vi "Run.vi"(8 "error in (no error)":errorcluster, 11 "Channel in":refnum<class "Channel.lvclass">) -> (0 "error out":errorcluster, 3 "Channel out":refnum<class "Channel.lvclass">)   [LabVIEW 2018, in "Channel.lvclass"]
uses:
  Channel.lvclass
  Channel.lvclass/Channel.ctl
  Simulated_Image_Constructor/Simulated_Image_Constructor.lvclass/Simulated_Image_Constructor.ctl
  State Machine/State Machine.lvclass/State Machine.ctl
  Save Image/Save Image.lvclass/Save Image.ctl
  Simulated_CCD_Camera/Simulated_CCD_Camera.lvclass/Simulated_CCD_Camera.ctl
  Simulated_Cooler/Simulated_Cooler.lvclass/Simulated_Cooler.ctl
  Simulated_CCD_Camera/Simulated_CCD_Camera.lvclass
  State Machine/State Machine.lvclass
  Simulated_Cooler/Simulated_Cooler.lvclass
  Save Image/Save Image.lvclass
  Interface/Interface.lvclass
  RxTx/RxTx.lvclass
  Simulated_Image_Constructor/Simulated_Image_Constructor.lvclass
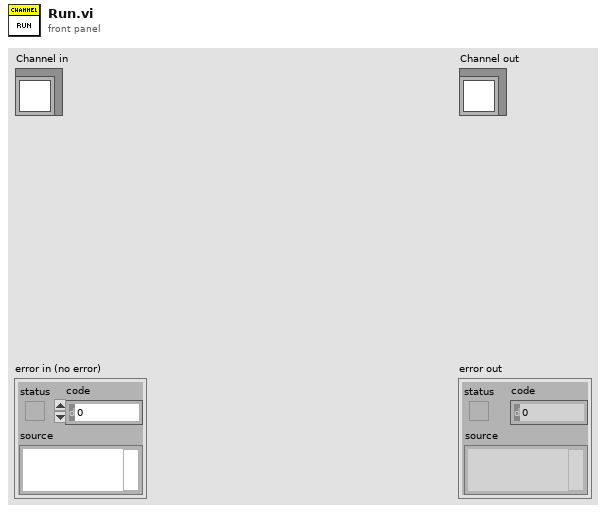
[diagram p1: front panel]
types:
  T1 = cluster{"Image Path":string, "Image Name":string, "Exposure Time":sgl, "Pre-amp gain":u8, "Readout Rate":u8, "EM Mode":u8, "EM Gain":u16, "Binning":u16, "Initial Line":u16, "Initial Cloumn":u16, "Final Line":u16, "Final Column":u16, "Kinetic Series Length":u32, "Shutter Mode":u8, "Cooler ON/OFF":u16, "Temperature":i8}
  T2 = cluster{"Exposure Time":sgl, "Pre-amp gain":u8, "Readout Rate":u8, "EM Mode":u8, "EM Gain":u16, "Binning":u16, "Initial Line":u16, "Initial Cloumn":u16, "Final Line":u16, "Final Column":u16, "Kinetic Series Length":u32, "Shutter Mode":u8, "Cooler ON/OFF":u8, "Temperature":i8, "Image Name":string, "Image Path":string, "Current Temperature":i16, "Temperatue Status":string, "Serial Number":u16, "#image":u32}
  T3 = cluster{"Exposure Time":sgl, "Pre-amp gain":u8, "Readout Rate":u8, "EM Mode":u8, "EM Gain":u16, "Binning":u16, "Initial Line":u16, "Initial Cloumn":u16, "Final Line":u16, "Final Column":u16, "Kinetic Series Length":u32, "Shutter Mode":u8, "Cooler ON/OFF":u16, "Temperature":i8, "Cubes":u32, "Trigger":u16}
  T4 = cluster{"Acquiring":bool, "Cube exposure time":sgl, "CCD status":string, "Frames done":u32, "Frame exposure time":dbl, "Initialization":bool, "Serial Number":u16}
  T5 = cluster{"Exposure Time":sgl, "EM Gain":u16, "Binning":u16, "Initial Line":u16, "Initial Cloumn":u16, "Final Line":u16, "Final Column":u16, "Kinetic Series Length":u32, "Shutter Mode":u8, "Pre-amp gain":u8, "Readout Rate":u8, "EM Mode":u8, "Trigger":u16, "Set Trigger":bool}
  T6 = cluster{"Initial Line":u16, "Initial Column":u16, "Final Line ":u16, "Final Column":u16, "Binning":u16, "Kinetic Series Length":u16, "Base Name":string, "Image Path":string}
  T7 = cluster{"Exposure Time":sgl, "Pre-amp gain":u8, "Readout Rate":u8, "EM Mode":u8, "EM Gain":u16, "Binning":u16, "Initial Line":u16, "Initial Cloumn":u16, "Final Line":u16, "Final Column":u16, "Kinetic Series Length":u32, "Shutter Mode":u8, "Cooler ON/OFF":u8, "Temperature":i8, "Image Name":string, "Image Path":string, "Current Temperature":i16, "Temperatue Status":string, "Serial Number":u16, " #image":u32}
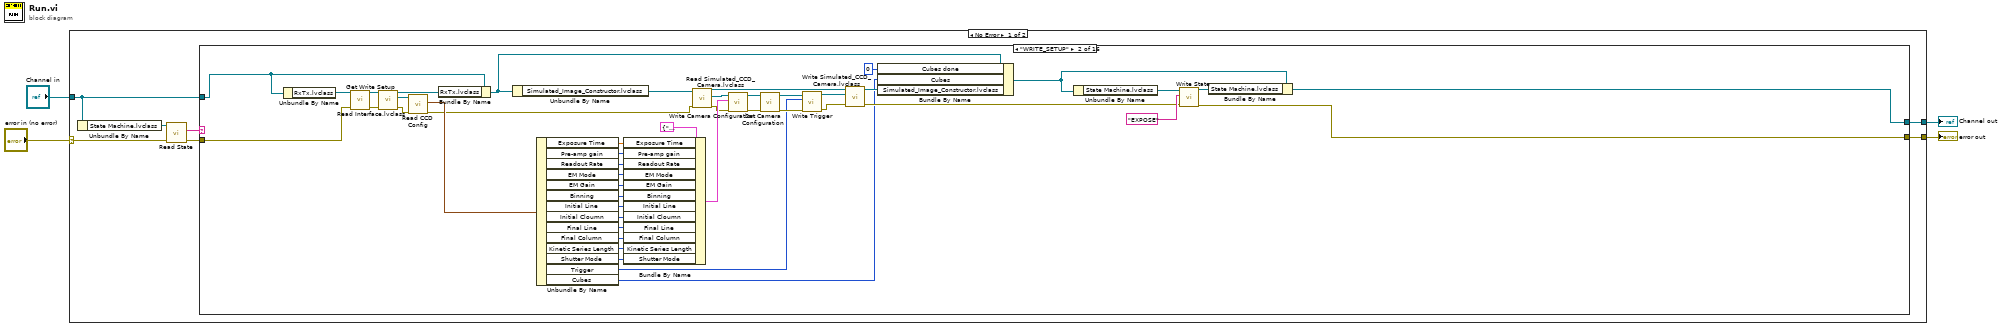
[diagram p0: block diagram]
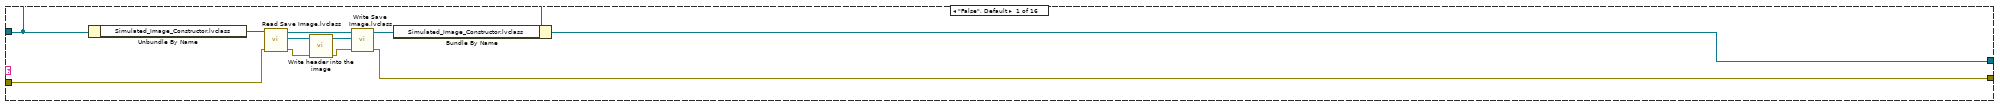
[diagram p2: hidden frame]
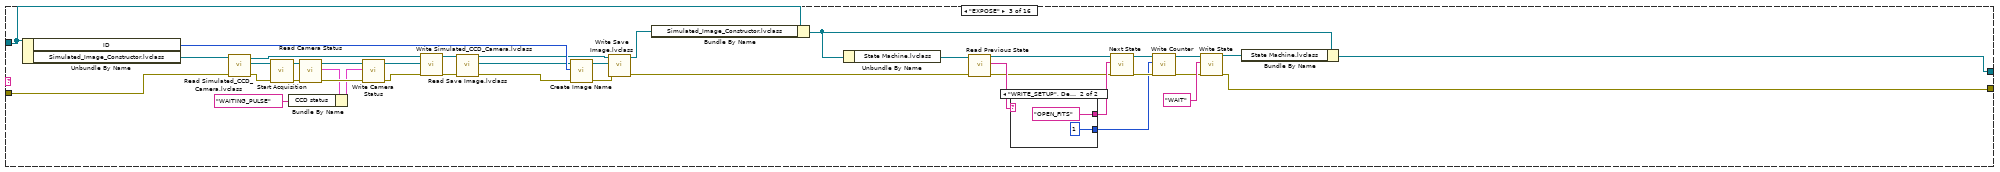
[diagram p3: hidden frame]
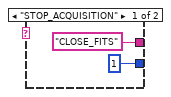
[diagram p4: hidden frame]
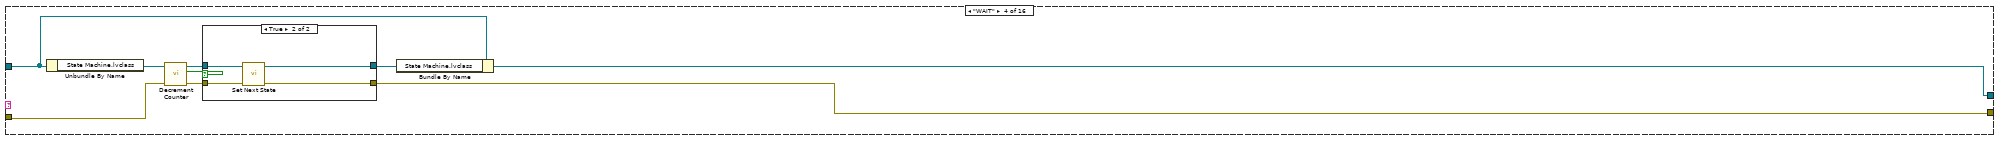
[diagram p5: hidden frame]
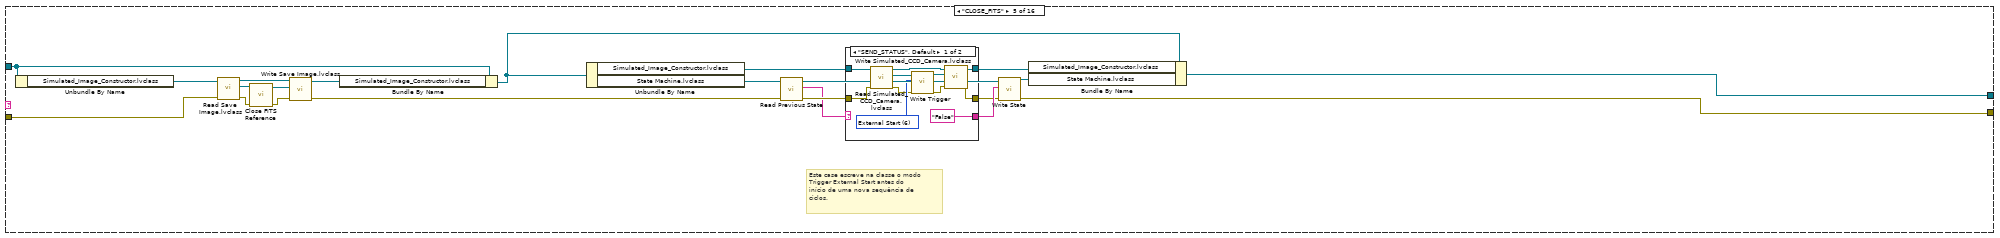
[diagram p7: hidden frame]
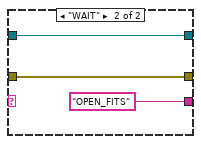
[diagram p8: hidden frame]
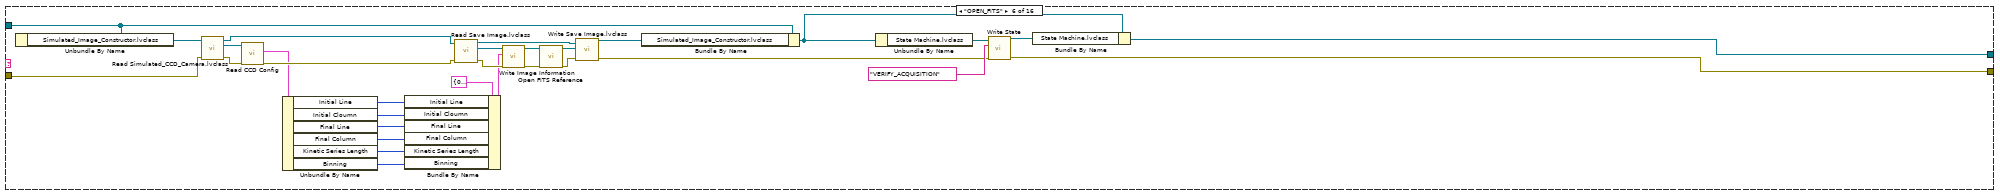
[diagram p9: hidden frame]
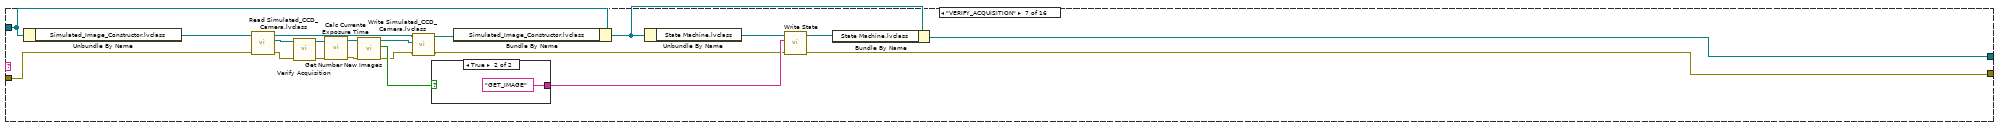
[diagram p10: hidden frame]
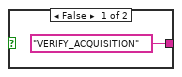
[diagram p11: hidden frame]
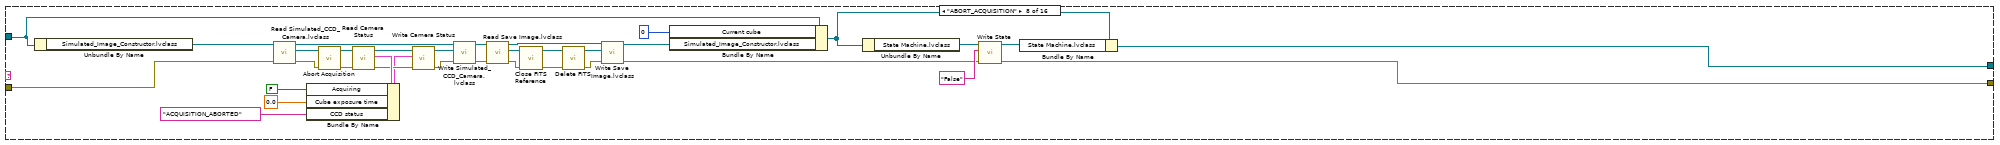
[diagram p12: hidden frame]
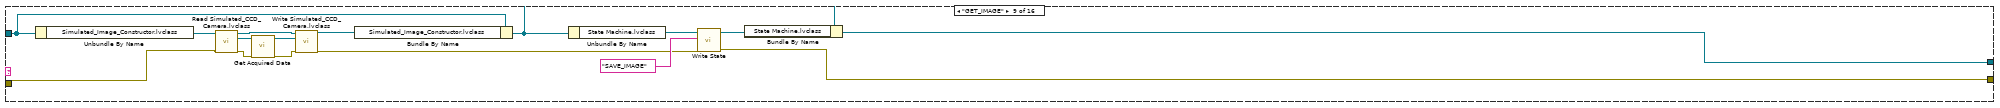
[diagram p13: hidden frame]
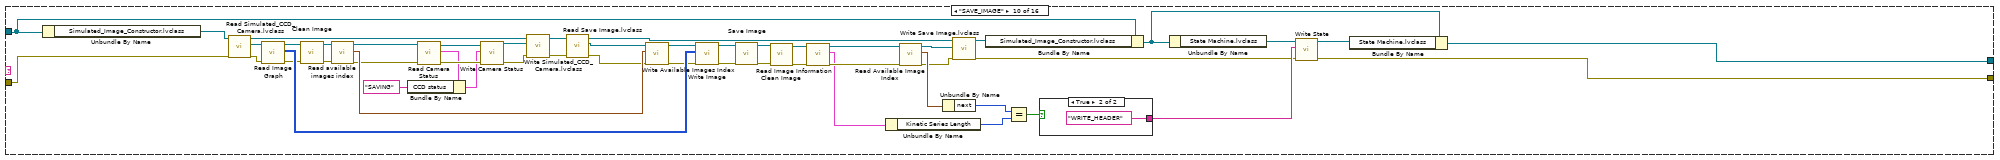
[diagram p14: hidden frame]
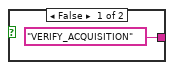
[diagram p15: hidden frame]
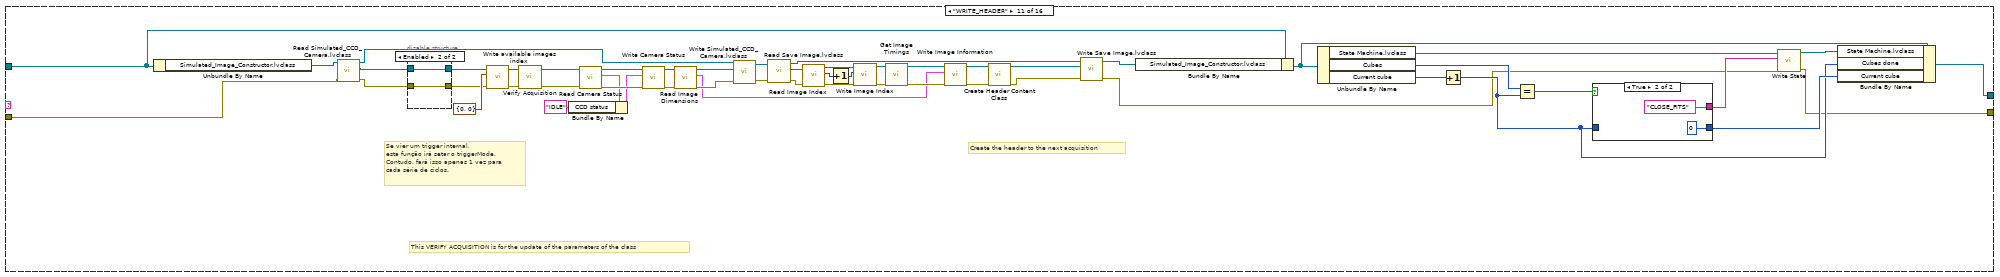
[diagram p16: hidden frame]
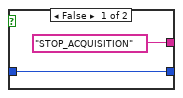
[diagram p17: hidden frame]
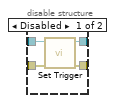
[diagram p18: hidden frame]
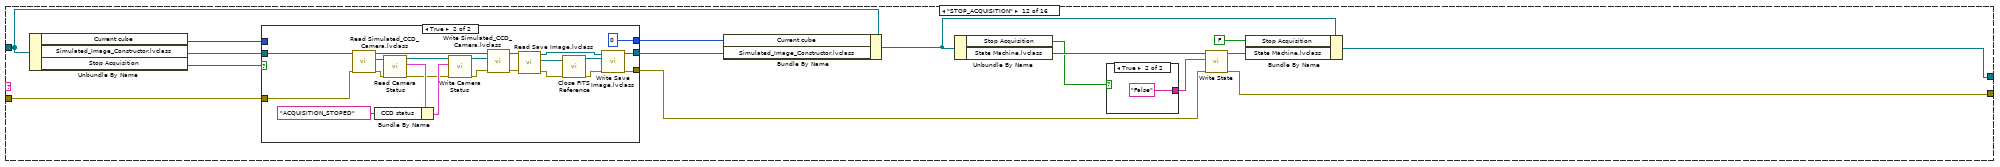
[diagram p19: hidden frame]
diagram:
  n1 = case shown="No Error" "error in (no error)" {
    selector: "error in (no error)" -> [w7 w1035]
    tunnel: [w11 w1035] -> w3
    tunnel: [w9 w1034] -> w1
    tunnel: "Channel in" -> [w10 w1034]
    frame No Error {
      n2 = Unbundle By Name(w10) -> ("State Machine.lvclass"=w8:refnum<class "State Machine.lvclass">)
      n3 = call-dynamic "Read State.vi"("error in (no error)"=w7, "State Machine in"=w8) -> ("error out"=w6:errorcluster, "State"=w5:string)  [unwired: 7 in, 1 out]
      n4 = case shown="\"WRITE_SETUP\"" w5 {
        tunnel: w6 -> [w14 w44 w83 w120 w130 w181 w202 w230 w259 w281 w346 w392 w428 w437 w836 w1017]
        tunnel: [w13 w39 w88 w117 w146 w190 w210 w248 w263 w296 w348 w396 w428 w430 w829 w1027] -> w11
        tunnel: [w21 w40 w85 w116 w148 w193 w213 w251 w268 w297 w349 w400 w429 w431 w830 w1028] -> w9
        tunnel: w10 -> [w22 w45 w108 w113 w149 w194 w215 w247 w267 w316 w373 w391 w429 w438 w837 w1033]
        frame "False", Default {
          n5 = Unbundle By Name(w22) -> ("Simulated_Image_Constructor.lvclass"=w20:refnum<class "Simulated_Image_Constructor.lvclass">)
          n6 = call "Read Save Image.lvclass.vi"("error in (no error)"=w14, "Image Constructor in"=w20) -> ("error out"=w16:errorcluster, "Save Image.lvclass"=w12:refnum<class "Save Image.lvclass">, "Image Constructor out"=w18:refnum<class "Simulated_Image_Constructor.lvclass">)  [unwired: 7 in]
          n7 = call "Write header into the image.vi"("error in (no error)"=w16, "Save Image in"=w12) -> ("error out"=w15:errorcluster, "Save Image out"=w19:refnum<class "Save Image.lvclass">)  [unwired: 8 in]
          n8 = call "Write Save Image.lvclass.vi"("error in (no error)"=w15, "Save Image.lvclass"=w19, "Image Constructor in"=w18) -> ("error out"=w13:errorcluster, "Image Constructor out"=w17:refnum<class "Simulated_Image_Constructor.lvclass">)  [unwired: 7 in]
          n9 = Bundle By Name(cluster=w22, "Simulated_Image_Constructor.lvclass"=w17) -> (w21:refnum<class "Channel.lvclass">)
        }
        frame "WRITE_SETUP" {
          n10 = Unbundle By Name(w45) -> ("RxTx.lvclass"=w62:refnum<class "RxTx.lvclass">)
          n11 = call "Get Write Setup.vi"("error in (no error)"=w44, "RxTx in"=w62) -> ("error out"=w63:errorcluster, "RxTx out"=w64:refnum<class "RxTx.lvclass">)  [unwired: 8 in]
          n12 = call "Read Interface.lvclass.vi"("error in (no error)"=w63, "RxTx in"=w64) -> ("error out"=w67:errorcluster, "Interface.lvclass"=w65:refnum<class "Interface.lvclass">, "RxTx out"=w66:refnum<class "RxTx.lvclass">)  [unwired: 7 in]
          n13 = call "Read CCD Config.vi"("error in (no error)"=w67, "Interface in"=w65) -> ("error out"=w31:errorcluster, "CCD Config"=w61:T3)  [unwired: 7 in, 1 out]
          n14 = Bundle By Name(cluster=w45, "RxTx.lvclass"=w66) -> (w60:refnum<class "Channel.lvclass">)
          n15 = Unbundle By Name(w60) -> ("Simulated_Image_Constructor.lvclass"=w30:refnum<class "Simulated_Image_Constructor.lvclass">)
          n16 = Unbundle By Name(w61) -> ("Exposure Time"=w35:sgl, "Pre-amp gain"=w49:u8, "Readout Rate"=w50:u8, "EM Mode"=w51:u8, "EM Gain"=w52:u16, "Binning"=w53:u16, "Initial Line"=w54:u16, "Initial Cloumn"=w55:u16, "Final Line"=w56:u16, "Final Column"=w57:u16, "Kinetic Series Length"=w34:u32, "Shutter Mode"=w58:u8, "Trigger"=w36:u16, "Cubes"=w24:u32)
          n17 = Bundle By Name(cluster=T1 {"Image Path"="", "Image Name"="Image", "Exposure Time"=0.1, "Pre-amp gain"=0, "Readout Rate"=0, "EM Mode"=0, "EM Gain"=2, "Binning"=1, "Initial Line"=1, "Initial Cloumn"=1, "Final Line"=1024, "Final Column"=1024, "Kinetic Series Length"=1, "Shutter Mode"=2, "Cooler ON/OFF"=0, "Temperature"=20} ("CCD Config"), "Exposure Time"=w35, "Pre-amp gain"=w49, "Readout Rate"=w50, "EM Mode"=w51, "EM Gain"=w52, "Binning"=w53, "Initial Line"=w54, "Initial Cloumn"=w55, "Final Line"=w56, "Final Column"=w57, "Kinetic Series Length"=w34, "Shutter Mode"=w58) -> (w59:T1)
          n18 = call "Read Simulated_CCD_Camera.lvclass.vi"("error in (no error)"=w31, "Image Constructor in"=w30) -> ("error out"=w32:errorcluster, "Simulated_CCD_Camera.lvclass"=w33:refnum<class "Simulated_CCD_Camera.lvclass">, "Image Constructor out"=w27:refnum<class "Simulated_Image_Constructor.lvclass">)  [unwired: 7 in]
          n19 = call-dynamic "Write Camera Configuration.vi"("error in (no error)"=w32, "CCD Config"=w59, "CCDCamera in"=w33) -> ("error out"=w47:errorcluster, "CCDCamera out"=w48:refnum<class "Simulated_CCD_Camera.lvclass">)  [unwired: 7 in]
          n20 = call-dynamic "Set Camera Configuration.vi"("error in (no error)"=w47, "CCDCamera in"=w48) -> ("error out"=w37:errorcluster, "CCDCamera out"=w38:refnum<class "Simulated_CCD_Camera.lvclass">)  [unwired: 8 in]
          n21 = call "Write Trigger.vi"("error in (no error)"=w37, "Trigger"=w36, "CCDCamera in"=w38) -> ("error out"=w29:errorcluster, "CCDCamera out"=w28:refnum<class "Simulated_CCD_Camera.lvclass">)  [unwired: 7 in]
          n22 = call "Write Simulated_CCD_Camera.lvclass.vi"("error in (no error)"=w29, "Simulated_CCD_Camera.lvclass"=w28, "Image Constructor in"=w27) -> ("error out"=w26:errorcluster, "Image Constructor out"=w25:refnum<class "Simulated_Image_Constructor.lvclass">)  [unwired: 7 in]
          n23 = Bundle By Name(cluster=w60, "Cubes done"=u16 0, "Cubes"=w24, "Simulated_Image_Constructor.lvclass"=w25) -> (w68:refnum<class "Channel.lvclass">)
          n24 = Unbundle By Name(w68) -> ("State Machine.lvclass"=w42:refnum<class "State Machine.lvclass">)
          n25 = call-dynamic "Write State.vi"("error in (no error)"=w26, "State"="EXPOSE", "State Machine in"=w42) -> ("error out"=w39:errorcluster, "State Machine out"=w43:refnum<class "State Machine.lvclass">)  [unwired: 7 in]
          n26 = Bundle By Name(cluster=w68, "State Machine.lvclass"=w43) -> (w40:refnum<class "Channel.lvclass">)
        }
        frame "EXPOSE" {
          n27 = Unbundle By Name(w108) -> ("ID"=w97:u8, "Simulated_Image_Constructor.lvclass"=w84:refnum<class "Simulated_Image_Constructor.lvclass">)
          n28 = call "Read Simulated_CCD_Camera.lvclass.vi"("error in (no error)"=w83, "Image Constructor in"=w84) -> ("error out"=w81:errorcluster, "Simulated_CCD_Camera.lvclass"=w82:refnum<class "Simulated_CCD_Camera.lvclass">, "Image Constructor out"=w80:refnum<class "Simulated_Image_Constructor.lvclass">)  [unwired: 7 in]
          n29 = call-dynamic "Start Acquisition.vi"("error in (no error)"=w81, "CCDCamera in"=w82) -> ("error out"=w106:errorcluster, "CCDCamera out"=w107:refnum<class "Simulated_CCD_Camera.lvclass">)  [unwired: 8 in]
          n30 = call "Read Camera Status.vi"("error in (no error)"=w106, "CCDCamera in"=w107) -> ("error out"=w104:errorcluster, "Camera Status"=w103:T4, "CCDCamera out"=w105:refnum<class "Simulated_CCD_Camera.lvclass">)  [unwired: 7 in]
          n31 = Bundle By Name(cluster=w103, "CCD status"="WAITING_PULSE" ("STATUS")) -> (w96:T4)
          n32 = call "Write Camera Status.vi"("error in (no error)"=w104, "Camera Status"=w96, "CCDCamera in"=w105) -> ("error out"=w71:errorcluster, "CCDCamera out"=w72:refnum<class "Simulated_CCD_Camera.lvclass">)  [unwired: 7 in]
          n33 = call "Write Simulated_CCD_Camera.lvclass.vi"("error in (no error)"=w71, "Simulated_CCD_Camera.lvclass"=w72, "Image Constructor in"=w80) -> ("error out"=w79:errorcluster, "Image Constructor out"=w78:refnum<class "Simulated_Image_Constructor.lvclass">)  [unwired: 7 in]
          n34 = call "Read Save Image.lvclass.vi"("error in (no error)"=w79, "Image Constructor in"=w78) -> ("error out"=w69:errorcluster, "Save Image.lvclass"=w70:refnum<class "Save Image.lvclass">, "Image Constructor out"=w75:refnum<class "Simulated_Image_Constructor.lvclass">)  [unwired: 7 in]
          n35 = call "Create Image Name.vi"("error in (no error)"=w69, "ID"=w97, "Save Image in"=w70) -> ("error out"=w77:errorcluster, "Save Image out"=w76:refnum<class "Save Image.lvclass">)  [unwired: 7 in]
          n36 = call "Write Save Image.lvclass.vi"("error in (no error)"=w77, "Save Image.lvclass"=w76, "Image Constructor in"=w75) -> ("error out"=w73:errorcluster, "Image Constructor out"=w74:refnum<class "Simulated_Image_Constructor.lvclass">)  [unwired: 7 in]
          n37 = Bundle By Name(cluster=w108, "Simulated_Image_Constructor.lvclass"=w74) -> (w86:refnum<class "Channel.lvclass">)
          n38 = Unbundle By Name(w86) -> ("State Machine.lvclass"=w101:refnum<class "State Machine.lvclass">)
          n39 = call-dynamic "Read Previous State.vi"("error in (no error)"=w73, "State Machine in"=w101) -> ("error out"=w99:errorcluster, "Previous State"=w100:string, "State Machine out"=w98:refnum<class "State Machine.lvclass">)  [unwired: 7 in]
          n40 = case shown="\"WRITE_SETUP\", Default" w100 {
            tunnel: ["CLOSE_FITS" "OPEN_FITS"] -> w102
            tunnel: [1 1] -> w89
            frame "STOP_ACQUISITION" {
            }
            frame "WRITE_SETUP", Default {
            }
          }
          n41 = call "Next State.vi"("error in (no error)"=w99, "New_State"=w102, "State Machine in"=w98) -> ("error out"=w90:errorcluster, "State Machine out"=w93:refnum<class "State Machine.lvclass">)  [unwired: 7 in]
          n42 = call "Write Counter.vi"("error in (no error)"=w90, "Counter"=w89, "State Machine in"=w93) -> ("error out"=w91:errorcluster, "State Machine out"=w92:refnum<class "State Machine.lvclass">)  [unwired: 7 in]
          n43 = call-dynamic "Write State.vi"("error in (no error)"=w91, "State"="WAIT", "State Machine in"=w92) -> ("error out"=w88:errorcluster, "State Machine out"=w87:refnum<class "State Machine.lvclass">)  [unwired: 7 in]
          n44 = Bundle By Name(cluster=w86, "State Machine.lvclass"=w87) -> (w85:refnum<class "Channel.lvclass">)
        }
        frame "WAIT" {
          n45 = Unbundle By Name(w113) -> ("State Machine.lvclass"=w121:refnum<class "State Machine.lvclass">)
          n46 = call "Decrement Counter.vi"("error in (no error)"=w120, "State Machine in"=w121) -> ("error out"=w118:errorcluster, "counter = zero"=w119:bool, "State Machine out"=w115:refnum<class "State Machine.lvclass">)  [unwired: 7 in]
          n47 = case shown="True" w119 {
            tunnel: w118 -> [w122 w127]
            tunnel: [w122 w125] -> w117
            tunnel: w115 -> [w123 w126]
            tunnel: [w123 w124] -> w114
            frame False {
            }
            frame True {
              n48 = call "Set Next State.vi"("error in (no error)"=w127, "State Machine in"=w126) -> ("error out"=w125:errorcluster, "State Machine out"=w124:refnum<class "State Machine.lvclass">)  [unwired: 8 in]
            }
          }
          n49 = Bundle By Name(cluster=w113, "State Machine.lvclass"=w114) -> (w116:refnum<class "Channel.lvclass">)
        }
        frame "CLOSE_FITS" {
          # "Este case escreve na classe o modo\nTrigger External Start antes do \ninício de uma nova sequência de \nciclos."
          n50 = Unbundle By Name(w149) -> ("Simulated_Image_Constructor.lvclass"=w133:refnum<class "Simulated_Image_Constructor.lvclass">)
          n51 = call "Read Save Image.lvclass.vi"("error in (no error)"=w130, "Image Constructor in"=w133) -> ("error out"=w137:errorcluster, "Save Image.lvclass"=w136:refnum<class "Save Image.lvclass">, "Image Constructor out"=w132:refnum<class "Simulated_Image_Constructor.lvclass">)  [unwired: 7 in]
          n52 = call "Close FITS Reference.vi"("error in (no error)"=w137, "Save Image in"=w136) -> ("error out"=w135:errorcluster, "Save Image out"=w134:refnum<class "Save Image.lvclass">)  [unwired: 8 in]
          n53 = call "Write Save Image.lvclass.vi"("error in (no error)"=w135, "Save Image.lvclass"=w134, "Image Constructor in"=w132) -> ("error out"=w128:errorcluster, "Image Constructor out"=w131:refnum<class "Simulated_Image_Constructor.lvclass">)  [unwired: 7 in]
          n54 = Bundle By Name(cluster=w149, "Simulated_Image_Constructor.lvclass"=w131) -> (w145:refnum<class "Channel.lvclass">)
          n55 = Unbundle By Name(w145) -> ("Simulated_Image_Constructor.lvclass"=w141:refnum<class "Simulated_Image_Constructor.lvclass">, "State Machine.lvclass"=w143:refnum<class "State Machine.lvclass">)
          n56 = call-dynamic "Read Previous State.vi"("error in (no error)"=w128, "State Machine in"=w143) -> ("error out"=w139:errorcluster, "Previous State"=w129:string, "State Machine out"=w142:refnum<class "State Machine.lvclass">)  [unwired: 7 in]
          n57 = case shown="\"SEND_STATUS\", Default" w129 {
            tunnel: ["False" "OPEN_FITS"] -> w144
            tunnel: w141 -> [w156 w162]
            tunnel: [w154 w162] -> w140
            tunnel: w139 -> [w155 w161]
            tunnel: [w153 w161] -> w138
            frame "SEND_STATUS", Default {
              w159 = u16 6 items=["Internal", "External", "-", "-", "-", "-", "External Start"] ("Trigger")
              n58 = call "Read Simulated_CCD_Camera.lvclass.vi"("error in (no error)"=w155, "Image Constructor in"=w156) -> ("error out"=w158:errorcluster, "Simulated_CCD_Camera.lvclass"=w157:refnum<class "Simulated_CCD_Camera.lvclass">, "Image Constructor out"=w150:refnum<class "Simulated_Image_Constructor.lvclass">)  [unwired: 7 in]
              n59 = call "Write Trigger.vi"("error in (no error)"=w158, "Trigger"=w159, "CCDCamera in"=w157) -> ("error out"=w152:errorcluster, "CCDCamera out"=w151:refnum<class "Simulated_CCD_Camera.lvclass">)  [unwired: 7 in]
              n60 = call "Write Simulated_CCD_Camera.lvclass.vi"("error in (no error)"=w152, "Simulated_CCD_Camera.lvclass"=w151, "Image Constructor in"=w150) -> ("error out"=w153:errorcluster, "Image Constructor out"=w154:refnum<class "Simulated_Image_Constructor.lvclass">)  [unwired: 7 in]
            }
            frame "WAIT" {
            }
          }
          n61 = call-dynamic "Write State.vi"("error in (no error)"=w138, "State"=w144, "State Machine in"=w142) -> ("error out"=w146:errorcluster, "State Machine out"=w147:refnum<class "State Machine.lvclass">)  [unwired: 7 in]
          n62 = Bundle By Name(cluster=w145, "Simulated_Image_Constructor.lvclass"=w140, "State Machine.lvclass"=w147) -> (w148:refnum<class "Channel.lvclass">)
        }
        frame "OPEN_FITS" {
          n63 = Unbundle By Name(w194) -> ("Simulated_Image_Constructor.lvclass"=w182:refnum<class "Simulated_Image_Constructor.lvclass">)
          n64 = call "Read Simulated_CCD_Camera.lvclass.vi"("error in (no error)"=w181, "Image Constructor in"=w182) -> ("error out"=w179:errorcluster, "Simulated_CCD_Camera.lvclass"=w180:refnum<class "Simulated_CCD_Camera.lvclass">, "Image Constructor out"=w178:refnum<class "Simulated_Image_Constructor.lvclass">)  [unwired: 7 in]
          n65 = call "Read CCD Config.vi"("error in (no error)"=w179, "CCDCamera in"=w180) -> ("error out"=w177:errorcluster, "CCD Config"=w170:T5)  [unwired: 7 in, 1 out]
          n66 = Unbundle By Name(w170) -> ("Initial Line"=w169:u16, "Initial Cloumn"=w168:u16, "Final Line"=w167:u16, "Final Column"=w166:u16, "Kinetic Series Length"=w165:u32, "Binning"=w164:u16)
          n67 = Bundle By Name(cluster=T2 {"Exposure Time"=0.0, "Pre-amp gain"=0, "Readout Rate"=0, "EM Mode"=0, "EM Gain"=2, "Binning"=1, "Initial Line"=1, "Initial Cloumn"=1, "Final Line"=1024, "Final Column"=1024, "Kinetic Series Length"=0, "Shutter Mode"=0, "Cooler ON/OFF"=0, "Temperature"=20, "Image Name"="", "Image Path"="", "Current Temperature"=0, "Temperatue Status"="", "Serial Number"=0, "#image"=0} ("CCD Config"), "Initial Line"=w169, "Initial Cloumn"=w168, "Final Line"=w167, "Final Column"=w166, "Kinetic Series Length"=w165, "Binning"=w164) -> (w172:T2)
          n68 = call "Read Save Image.lvclass.vi"("error in (no error)"=w177, "Image Constructor in"=w178) -> ("error out"=w173:errorcluster, "Save Image.lvclass"=w174:refnum<class "Save Image.lvclass">, "Image Constructor out"=w185:refnum<class "Simulated_Image_Constructor.lvclass">)  [unwired: 7 in]
          n69 = call "Write Image Information.vi"("error in (no error)"=w173, "CCD Config"=w172, "Save Image in"=w174) -> ("error out"=w176:errorcluster, "Save Image out"=w175:refnum<class "Save Image.lvclass">)  [unwired: 7 in]
          n70 = call "Open FITS Reference.vi"("error in (no error)"=w176, "Save Image in"=w175) -> ("error out"=w187:errorcluster, "Save Image out"=w186:refnum<class "Save Image.lvclass">)  [unwired: 8 in]
          n71 = call "Write Save Image.lvclass.vi"("error in (no error)"=w187, "Save Image.lvclass"=w186, "Image Constructor in"=w185) -> ("error out"=w183:errorcluster, "Image Constructor out"=w184:refnum<class "Simulated_Image_Constructor.lvclass">)  [unwired: 7 in]
          n72 = Bundle By Name(cluster=w194, "Simulated_Image_Constructor.lvclass"=w184) -> (w189:refnum<class "Channel.lvclass">)
          n73 = Unbundle By Name(w189) -> ("State Machine.lvclass"=w191:refnum<class "State Machine.lvclass">)
          n74 = call-dynamic "Write State.vi"("error in (no error)"=w183, "State"="VERIFY_ACQUISITION", "State Machine in"=w191) -> ("error out"=w190:errorcluster, "State Machine out"=w192:refnum<class "State Machine.lvclass">)  [unwired: 7 in]
          n75 = Bundle By Name(cluster=w189, "State Machine.lvclass"=w192) -> (w193:refnum<class "Channel.lvclass">)
        }
        frame "VERIFY_ACQUISITION" {
          n76 = Unbundle By Name(w215) -> ("Simulated_Image_Constructor.lvclass"=w203:refnum<class "Simulated_Image_Constructor.lvclass">)
          n77 = call "Read Simulated_CCD_Camera.lvclass.vi"("error in (no error)"=w202, "Image Constructor in"=w203) -> ("error out"=w200:errorcluster, "Simulated_CCD_Camera.lvclass"=w201:refnum<class "Simulated_CCD_Camera.lvclass">, "Image Constructor out"=w198:refnum<class "Simulated_Image_Constructor.lvclass">)  [unwired: 7 in]
          n78 = call-dynamic "Verify Acquisition.vi"("error in (no error)"=w200, "CCDCamera in"=w201) -> ("error out"=w204:errorcluster, "CCDCamera out"=w205:refnum<class "Simulated_CCD_Camera.lvclass">)  [unwired: 7 in, 1 out]
          n79 = call-dynamic "Calc Currente Exposure Time.vi"("error in (no error)"=w204, "CCDCamera in"=w205) -> ("error out"=w206:errorcluster, "CCDCamera out"=w207:refnum<class "Simulated_CCD_Camera.lvclass">)  [unwired: 8 in]
          n80 = call-dynamic "Get Number New Images.vi"("error in (no error)"=w206, "CCDCamera in"=w207) -> ("error out"=w196:errorcluster, "New Images ?"=w208:bool, "CCDCamera out"=w195:refnum<class "Simulated_CCD_Camera.lvclass">)  [unwired: 7 in]
          n81 = call "Write Simulated_CCD_Camera.lvclass.vi"("error in (no error)"=w196, "Simulated_CCD_Camera.lvclass"=w195, "Image Constructor in"=w198) -> ("error out"=w197:errorcluster, "Image Constructor out"=w199:refnum<class "Simulated_Image_Constructor.lvclass">)  [unwired: 7 in]
          n82 = case shown="True" w208 {
            tunnel: ["VERIFY_ACQUISITION" "GET_IMAGE"] -> w209
            frame False {
            }
            frame True {
            }
          }
          n83 = Bundle By Name(cluster=w215, "Simulated_Image_Constructor.lvclass"=w199) -> (w214:refnum<class "Channel.lvclass">)
          n84 = Unbundle By Name(w214) -> ("State Machine.lvclass"=w212:refnum<class "State Machine.lvclass">)
          n85 = call-dynamic "Write State.vi"("error in (no error)"=w197, "State"=w209, "State Machine in"=w212) -> ("error out"=w210:errorcluster, "State Machine out"=w211:refnum<class "State Machine.lvclass">)  [unwired: 7 in]
          n86 = Bundle By Name(cluster=w214, "State Machine.lvclass"=w211) -> (w213:refnum<class "Channel.lvclass">)
        }
        frame "ABORT_ACQUISITION" {
          n87 = Unbundle By Name(w247) -> ("Simulated_Image_Constructor.lvclass"=w231:refnum<class "Simulated_Image_Constructor.lvclass">)
          n88 = call "Read Simulated_CCD_Camera.lvclass.vi"("error in (no error)"=w230, "Image Constructor in"=w231) -> ("error out"=w232:errorcluster, "Simulated_CCD_Camera.lvclass"=w233:refnum<class "Simulated_CCD_Camera.lvclass">, "Image Constructor out"=w227:refnum<class "Simulated_Image_Constructor.lvclass">)  [unwired: 7 in]
          n89 = call-dynamic "Abort Acquisition.vi"("error in (no error)"=w232, "CCDCamera in"=w233) -> ("error out"=w239:errorcluster, "CCDCamera out"=w240:refnum<class "Simulated_CCD_Camera.lvclass">)  [unwired: 8 in]
          n90 = call "Read Camera Status.vi"("error in (no error)"=w239, "CCDCamera in"=w240) -> ("error out"=w237:errorcluster, "Camera Status"=w244:T4, "CCDCamera out"=w238:refnum<class "Simulated_CCD_Camera.lvclass">)  [unwired: 7 in]
          n91 = Bundle By Name(cluster=w244, "Acquiring"=FALSE, "Cube exposure time"=sgl 0.0 ("Current exptime"), "CCD status"="ACQUISITION_ABORTED" ("STATUS")) -> (w236:T4)
          n92 = call "Write Camera Status.vi"("error in (no error)"=w237, "Camera Status"=w236, "CCDCamera in"=w238) -> ("error out"=w229:errorcluster, "CCDCamera out"=w228:refnum<class "Simulated_CCD_Camera.lvclass">)  [unwired: 7 in]
          n93 = call "Write Simulated_CCD_Camera.lvclass.vi"("error in (no error)"=w229, "Simulated_CCD_Camera.lvclass"=w228, "Image Constructor in"=w227) -> ("error out"=w226:errorcluster, "Image Constructor out"=w225:refnum<class "Simulated_Image_Constructor.lvclass">)  [unwired: 7 in]
          n94 = call "Read Save Image.lvclass.vi"("error in (no error)"=w226, "Image Constructor in"=w225) -> ("error out"=w224:errorcluster, "Save Image.lvclass"=w223:refnum<class "Save Image.lvclass">, "Image Constructor out"=w221:refnum<class "Simulated_Image_Constructor.lvclass">)  [unwired: 7 in]
          n95 = call "Close FITS Reference.vi"("error in (no error)"=w224, "Save Image in"=w223) -> ("error out"=w234:errorcluster, "Save Image out"=w235:refnum<class "Save Image.lvclass">)  [unwired: 8 in]
          n96 = call "Delete FITS.vi"("error in (no error)"=w234, "Save Image in"=w235) -> ("error out"=w220:errorcluster, "Save Image out"=w222:refnum<class "Save Image.lvclass">)  [unwired: 8 in]
          n97 = call "Write Save Image.lvclass.vi"("error in (no error)"=w220, "Save Image.lvclass"=w222, "Image Constructor in"=w221) -> ("error out"=w218:errorcluster, "Image Constructor out"=w219:refnum<class "Simulated_Image_Constructor.lvclass">)  [unwired: 7 in]
          n98 = Bundle By Name(cluster=w247, "Current cube"=0, "Simulated_Image_Constructor.lvclass"=w219) -> (w252:refnum<class "Channel.lvclass">)
          n99 = Unbundle By Name(w252) -> ("State Machine.lvclass"=w250:refnum<class "State Machine.lvclass">)
          n100 = call-dynamic "Write State.vi"("error in (no error)"=w218, "State"="False", "State Machine in"=w250) -> ("error out"=w248:errorcluster, "State Machine out"=w249:refnum<class "State Machine.lvclass">)  [unwired: 7 in]
          n101 = Bundle By Name(cluster=w252, "State Machine.lvclass"=w249) -> (w251:refnum<class "Channel.lvclass">)
        }
        frame "GET_IMAGE" {
          n102 = Unbundle By Name(w267) -> ("Simulated_Image_Constructor.lvclass"=w260:refnum<class "Simulated_Image_Constructor.lvclass">)
          n103 = call "Read Simulated_CCD_Camera.lvclass.vi"("error in (no error)"=w259, "Image Constructor in"=w260) -> ("error out"=w258:errorcluster, "Simulated_CCD_Camera.lvclass"=w261:refnum<class "Simulated_CCD_Camera.lvclass">, "Image Constructor out"=w256:refnum<class "Simulated_Image_Constructor.lvclass">)  [unwired: 7 in]
          n104 = call-dynamic "Get Acquired Data.vi"("error in (no error)"=w258, "CCDCamera in"=w261) -> ("error out"=w254:errorcluster, "CCDCamera out"=w255:refnum<class "Simulated_CCD_Camera.lvclass">)  [unwired: 8 in]
          n105 = call "Write Simulated_CCD_Camera.lvclass.vi"("error in (no error)"=w254, "Simulated_CCD_Camera.lvclass"=w255, "Image Constructor in"=w256) -> ("error out"=w253:errorcluster, "Image Constructor out"=w257:refnum<class "Simulated_Image_Constructor.lvclass">)  [unwired: 7 in]
          n106 = Bundle By Name(cluster=w267, "Simulated_Image_Constructor.lvclass"=w257) -> (w266:refnum<class "Channel.lvclass">)
          n107 = Unbundle By Name(w266) -> ("State Machine.lvclass"=w264:refnum<class "State Machine.lvclass">)
          n108 = call-dynamic "Write State.vi"("error in (no error)"=w253, "State"="SAVE_IMAGE", "State Machine in"=w264) -> ("error out"=w263:errorcluster, "State Machine out"=w265:refnum<class "State Machine.lvclass">)  [unwired: 7 in]
          n109 = Bundle By Name(cluster=w266, "State Machine.lvclass"=w265) -> (w268:refnum<class "Channel.lvclass">)
        }
        frame "SAVE_IMAGE" {
          n110 = Unbundle By Name(w316) -> ("Simulated_Image_Constructor.lvclass"=w282:refnum<class "Simulated_Image_Constructor.lvclass">)
          n111 = call "Read Simulated_CCD_Camera.lvclass.vi"("error in (no error)"=w281, "Image Constructor in"=w282) -> ("error out"=w284:errorcluster, "Simulated_CCD_Camera.lvclass"=w283:refnum<class "Simulated_CCD_Camera.lvclass">, "Image Constructor out"=w280:refnum<class "Simulated_Image_Constructor.lvclass">)  [unwired: 7 in]
          n112 = call "Read Image Graph.vi"("error in (no error)"=w284, "CCDCamera in"=w283) -> ("error out"=w317:errorcluster, "Image Graph"=w319:u16[][][], "CCDCamera out"=w318:refnum<class "Simulated_CCD_Camera.lvclass">)  [unwired: 7 in]
          n113 = call "Clean Image.vi"("error in (no error)"=w317, "CCDCamera in"=w318) -> ("error out"=w310:errorcluster, "CCDCamera out"=w311:refnum<class "Simulated_CCD_Camera.lvclass">)  [unwired: 8 in]
          n114 = call "Read available images index.vi"("error in (no error)"=w310, "CCDCamera in"=w311) -> ("error out"=w287:errorcluster, "available images index"=w295:cluster{"previous":u16, "next":u16}, "CCDCamera out"=w289:refnum<class "Simulated_CCD_Camera.lvclass">)  [unwired: 7 in]
          n115 = call "Read Camera Status.vi"("error in (no error)"=w287, "CCDCamera in"=w289) -> ("error out"=w291:errorcluster, "Camera Status"=w286:T4, "CCDCamera out"=w288:refnum<class "Simulated_CCD_Camera.lvclass">)  [unwired: 7 in]
          n116 = Bundle By Name(cluster=w286, "CCD status"="SAVING" ("STATUS")) -> (w285:T4)
          n117 = call "Write Camera Status.vi"("error in (no error)"=w291, "Camera Status"=w285, "CCDCamera in"=w288) -> ("error out"=w278:errorcluster, "CCDCamera out"=w279:refnum<class "Simulated_CCD_Camera.lvclass">)  [unwired: 7 in]
          n118 = call "Write Simulated_CCD_Camera.lvclass.vi"("error in (no error)"=w278, "Simulated_CCD_Camera.lvclass"=w279, "Image Constructor in"=w280) -> ("error out"=w277:errorcluster, "Image Constructor out"=w276:refnum<class "Simulated_Image_Constructor.lvclass">)  [unwired: 7 in]
          n119 = call "Read Save Image.lvclass.vi"("error in (no error)"=w277, "Image Constructor in"=w276) -> ("error out"=w275:errorcluster, "Save Image.lvclass"=w274:refnum<class "Save Image.lvclass">, "Image Constructor out"=w271:refnum<class "Simulated_Image_Constructor.lvclass">)  [unwired: 7 in]
          n120 = call "Write Available Images Index.vi"("error in (no error)"=w275, "available images index"=w295, "Save Image in"=w274) -> ("error out"=w309:errorcluster, "Save Image out"=w308:refnum<class "Save Image.lvclass">)  [unwired: 7 in]
          n121 = call "Write Image.vi"("error in (no error)"=w309, "Image"=w319, "Save Image in"=w308) -> ("error out"=w312:errorcluster, "Save Image out"=w313:refnum<class "Save Image.lvclass">)  [unwired: 7 in]
          n122 = call "Save Image.vi"("error in (no error)"=w312, "Save Image in"=w313) -> ("error out"=w314:errorcluster, "Save Image out"=w315:refnum<class "Save Image.lvclass">)  [unwired: 8 in]
          n123 = call "Clean Image.vi"("error in (no error)"=w314, "Save Image in"=w315) -> ("error out"=w307:errorcluster, "Save Image out"=w306:refnum<class "Save Image.lvclass">)  [unwired: 8 in]
          n124 = call "Read Image Information.vi"("error in (no error)"=w307, "Save Image in"=w306) -> ("error out"=w305:errorcluster, "Image Information"=w304:T6, "Save Image out"=w292:refnum<class "Save Image.lvclass">)  [unwired: 7 in]
          n125 = Unbundle By Name(w304) -> ("Kinetic Series Length"=w303:u16)
          n126 = call "Read Available Image Index.vi"("error in (no error)"=w305, "Save Image in"=w292) -> ("error out"=w272:errorcluster, "available images index"=w294:cluster{"previous":u16, "next":u16}, "Save Image out"=w270:refnum<class "Save Image.lvclass">)  [unwired: 7 in]
          n127 = Unbundle By Name(w294) -> ("next"=w293:u16)
          n128 = call "Write Save Image.lvclass.vi"("error in (no error)"=w272, "Save Image.lvclass"=w270, "Image Constructor in"=w271) -> ("error out"=w269:errorcluster, "Image Constructor out"=w273:refnum<class "Simulated_Image_Constructor.lvclass">)  [unwired: 7 in]
          n129 = Bundle By Name(cluster=w316, "Simulated_Image_Constructor.lvclass"=w273) -> (w299:refnum<class "Channel.lvclass">)
          n130 = Equal?(x=w293, y=w303) -> (x = y?=w302:bool)
          n131 = case shown="True" w302 {
            tunnel: ["VERIFY_ACQUISITION" "WRITE_HEADER"] -> w300
            frame False {
            }
            frame True {
            }
          }
          n132 = Unbundle By Name(w299) -> ("State Machine.lvclass"=w301:refnum<class "State Machine.lvclass">)
          n133 = call-dynamic "Write State.vi"("error in (no error)"=w269, "State"=w300, "State Machine in"=w301) -> ("error out"=w296:errorcluster, "State Machine out"=w298:refnum<class "State Machine.lvclass">)  [unwired: 7 in]
          n134 = Bundle By Name(cluster=w299, "State Machine.lvclass"=w298) -> (w297:refnum<class "Channel.lvclass">)
        }
        frame "WRITE_HEADER" {
          # "Create the header to the next acquisition"
          # "Se vier um trigger internal, \nesta função irá setar o triggerMode.\nContudo, fará isso apenas 1 vez para\ncada série de ciclos."
          # "This VERIFY ACQUISITION is for the update of the parameters of the class"
          n135 = Unbundle By Name(w373) -> ("Simulated_Image_Constructor.lvclass"=w347:refnum<class "Simulated_Image_Constructor.lvclass">)
          n136 = call "Read Simulated_CCD_Camera.lvclass.vi"("error in (no error)"=w346, "Image Constructor in"=w347) -> ("error out"=w361:errorcluster, "Simulated_CCD_Camera.lvclass"=w360:refnum<class "Simulated_CCD_Camera.lvclass">, "Image Constructor out"=w359:refnum<class "Simulated_Image_Constructor.lvclass">)  [unwired: 7 in]
          n137 = disable-structure shown="Enabled" {
            disable-tunnel: [w382 w384] -> w363
            disable-tunnel: [w381 w383] -> w362
            disable-tunnel: w360 -> [w380 w384]
            disable-tunnel: w361 -> [w379 w383]
            frame Disabled {
              n138 = call-dynamic "Set Trigger.vi"("error in (no error)"=w379, "CCDCamera in"=w380) -> ("error out"=w381:errorcluster, "CCDCamera out"=w382:refnum<class "Simulated_CCD_Camera.lvclass">)  [unwired: 8 in]
            }
            frame Enabled {
            }
          }
          n139 = call "Write available images index.vi"("error in (no error)"=w362, "available images index"=cluster{"previous":u16, "next":u16} {"previous"=0, "next"=0}, "CCDCamera in"=w363) -> ("error out"=w371:errorcluster, "CCDCamera out"=w372:refnum<class "Simulated_CCD_Camera.lvclass">)  [unwired: 7 in]
          n140 = call-dynamic "Verify Acquisition.vi"("error in (no error)"=w371, "CCDCamera in"=w372) -> ("error out"=w365:errorcluster, "CCDCamera out"=w366:refnum<class "Simulated_CCD_Camera.lvclass">)  [unwired: 7 in, 1 out]
          n141 = call "Read Camera Status.vi"("error in (no error)"=w365, "CCDCamera in"=w366) -> ("error out"=w369:errorcluster, "Camera Status"=w368:T4, "CCDCamera out"=w370:refnum<class "Simulated_CCD_Camera.lvclass">)  [unwired: 7 in]
          n142 = Bundle By Name(cluster=w368, "CCD status"="IDLE" ("STATUS")) -> (w367:T4)
          n143 = call "Write Camera Status.vi"("error in (no error)"=w369, "Camera Status"=w367, "CCDCamera in"=w370) -> ("error out"=w331:errorcluster, "CCDCamera out"=w332:refnum<class "Simulated_CCD_Camera.lvclass">)  [unwired: 7 in]
          n144 = call "Read Image Dimensions.vi"("error in (no error)"=w331, "CCDCamera in"=w332) -> ("error out"=w330:errorcluster, "CCD Config"=w326:T7, "CCDCamera out"=w329:refnum<class "Simulated_CCD_Camera.lvclass">)  [unwired: 7 in]
          n145 = call "Write Simulated_CCD_Camera.lvclass.vi"("error in (no error)"=w330, "Simulated_CCD_Camera.lvclass"=w329, "Image Constructor in"=w359) -> ("error out"=w335:errorcluster, "Image Constructor out"=w336:refnum<class "Simulated_Image_Constructor.lvclass">)  [unwired: 7 in]
          n146 = call "Read Save Image.lvclass.vi"("error in (no error)"=w335, "Image Constructor in"=w336) -> ("error out"=w339:errorcluster, "Save Image.lvclass"=w338:refnum<class "Save Image.lvclass">, "Image Constructor out"=w337:refnum<class "Simulated_Image_Constructor.lvclass">)  [unwired: 7 in]
          n147 = call "Read Image Index.vi"("error in (no error)"=w339, "Save Image in"=w338) -> ("error out"=w342:errorcluster, "Image Index"=w341:u16, "Save Image out"=w343:refnum<class "Save Image.lvclass">)  [unwired: 7 in]
          n148 = Increment(x=w341) -> (x+1=w340:u16)
          n149 = call "Write Image Index.vi"("error in (no error)"=w342, "Image Index"=w340, "Save Image in"=w343) -> ("error out"=w344:errorcluster, "Save Image out"=w345:refnum<class "Save Image.lvclass">)  [unwired: 7 in]
          n150 = call "Get Image Timings.vi"("error in (no error)"=w344, "Save Image in"=w345) -> ("error out"=w327:errorcluster, "Save Image out"=w328:refnum<class "Save Image.lvclass">)  [unwired: 8 in]
          n151 = call "Write Image Information.vi"("error in (no error)"=w327, "CCD Config"=w326, "Save Image in"=w328) -> ("error out"=w325:errorcluster, "Save Image out"=w323:refnum<class "Save Image.lvclass">)  [unwired: 7 in]
          n152 = call "Create Header Content Class.vi"("error in (no error)"=w325, "Save Image in"=w323) -> ("error out"=w324:errorcluster, "Save Image out"=w322:refnum<class "Save Image.lvclass">)  [unwired: 8 in]
          n153 = call "Write Save Image.lvclass.vi"("error in (no error)"=w324, "Save Image.lvclass"=w322, "Image Constructor in"=w337) -> ("error out"=w333:errorcluster, "Image Constructor out"=w334:refnum<class "Simulated_Image_Constructor.lvclass">)  [unwired: 7 in]
          n154 = Bundle By Name(cluster=w373, "Simulated_Image_Constructor.lvclass"=w334) -> (w350:refnum<class "Channel.lvclass">)
          n155 = Unbundle By Name(w350) -> ("State Machine.lvclass"=w354:refnum<class "State Machine.lvclass">, "Cubes"=w356:u16, "Current cube"=w353:u16)
          n156 = Increment(x=w353) -> (x+1=w351:u16)
          n157 = Equal?(x=w356, y=w351) -> (x = y?=w355:bool)
          n158 = case shown="True" w355 {
            tunnel: ["STOP_ACQUISITION" "CLOSE_FITS"] -> w357
            tunnel: [w375 u16 0 ("current image")] -> w352
            tunnel: w351 -> [w375 _]
            frame False {
            }
            frame True {
            }
          }
          n159 = call-dynamic "Write State.vi"("error in (no error)"=w333, "State"=w357, "State Machine in"=w354) -> ("error out"=w348:errorcluster, "State Machine out"=w358:refnum<class "State Machine.lvclass">)  [unwired: 7 in]
          n160 = Bundle By Name(cluster=w350, "State Machine.lvclass"=w358, "Cubes done"=w351, "Current cube"=w352) -> (w349:refnum<class "Channel.lvclass">)
        }
        frame "STOP_ACQUISITION" {
          n161 = Unbundle By Name(w391) -> ("Current cube"=w386:u16, "Simulated_Image_Constructor.lvclass"=w393:refnum<class "Simulated_Image_Constructor.lvclass">, "Stop Acquisition"=w387:bool)
          n162 = case shown="True" w387 {
            tunnel: w393 -> [w403 w417]
            tunnel: w392 -> [w402 w416]
            tunnel: [w403 w405] -> w390
            tunnel: [w402 w404] -> w388
            tunnel: w386 -> [w401 _]
            tunnel: [w401 0] -> w385
            frame False {
            }
            frame True {
              n163 = call "Read Simulated_CCD_Camera.lvclass.vi"("error in (no error)"=w416, "Image Constructor in"=w417) -> ("error out"=w419:errorcluster, "Simulated_CCD_Camera.lvclass"=w418:refnum<class "Simulated_CCD_Camera.lvclass">, "Image Constructor out"=w413:refnum<class "Simulated_Image_Constructor.lvclass">)  [unwired: 7 in]
              n164 = call "Read Camera Status.vi"("error in (no error)"=w419, "CCDCamera in"=w418) -> ("error out"=w423:errorcluster, "Camera Status"=w425:T4, "CCDCamera out"=w422:refnum<class "Simulated_CCD_Camera.lvclass">)  [unwired: 7 in]
              n165 = Bundle By Name(cluster=w425, "CCD status"="ACQUISITION_STOPED") -> (w424:T4)
              n166 = call "Write Camera Status.vi"("error in (no error)"=w423, "Camera Status"=w424, "CCDCamera in"=w422) -> ("error out"=w415:errorcluster, "CCDCamera out"=w414:refnum<class "Simulated_CCD_Camera.lvclass">)  [unwired: 7 in]
              n167 = call "Write Simulated_CCD_Camera.lvclass.vi"("error in (no error)"=w415, "Simulated_CCD_Camera.lvclass"=w414, "Image Constructor in"=w413) -> ("error out"=w412:errorcluster, "Image Constructor out"=w411:refnum<class "Simulated_Image_Constructor.lvclass">)  [unwired: 7 in]
              n168 = call "Read Save Image.lvclass.vi"("error in (no error)"=w412, "Image Constructor in"=w411) -> ("error out"=w409:errorcluster, "Save Image.lvclass"=w410:refnum<class "Save Image.lvclass">, "Image Constructor out"=w406:refnum<class "Simulated_Image_Constructor.lvclass">)  [unwired: 7 in]
              n169 = call "Close FITS Reference.vi"("error in (no error)"=w409, "Save Image in"=w410) -> ("error out"=w408:errorcluster, "Save Image out"=w407:refnum<class "Save Image.lvclass">)  [unwired: 8 in]
              n170 = call "Write Save Image.lvclass.vi"("error in (no error)"=w408, "Save Image.lvclass"=w407, "Image Constructor in"=w406) -> ("error out"=w404:errorcluster, "Image Constructor out"=w405:refnum<class "Simulated_Image_Constructor.lvclass">)  [unwired: 7 in]
            }
          }
          n171 = Bundle By Name(cluster=w391, "Current cube"=w385, "Simulated_Image_Constructor.lvclass"=w390) -> (w389:refnum<class "Channel.lvclass">)
          n172 = Unbundle By Name(w389) -> ("Stop Acquisition"=w395:bool, "State Machine.lvclass"=w398:refnum<class "State Machine.lvclass">)
          n173 = case shown="True" w395 {
            tunnel: ["EXPOSE" "False"] -> w394
            frame False {
            }
            frame True {
            }
          }
          n174 = call-dynamic "Write State.vi"("error in (no error)"=w388, "State"=w394, "State Machine in"=w398) -> ("error out"=w396:errorcluster, "State Machine out"=w397:refnum<class "State Machine.lvclass">)  [unwired: 7 in]
          n175 = Bundle By Name(cluster=w389, "Stop Acquisition"=FALSE, "State Machine.lvclass"=w397) -> (w400:refnum<class "Channel.lvclass">)
        }
        frame "N/A" {
        }
        frame "SET" {
          n176 = Unbundle By Name(w438) -> ("RxTx.lvclass"=w444:refnum<class "RxTx.lvclass">)
          n177 = call "Read Rx Value.vi"("error in (no error)"=w437, "RxTx in"=w444) -> ("error out"=w446:errorcluster, "Rx value"=w445:string, "RxTx out"=w447:refnum<class "RxTx.lvclass">)  [unwired: 7 in]
          n178 = case shown="\"READOUT\"" w445 {
            tunnel: [w450 w462 w490 w518 w541 w561 w582 w602 w620 w638 w649 w671 w686 w703 w718 w733 w756 w775 w796 w814 w816 w823] -> w443
            tunnel: w438 -> [w450 w463 w489 w517 w540 w560 w581 w601 w619 w637 w650 w670 w685 w702 w717 w732 w755 w774 w795 w813 w820 w823]
            tunnel: [w449 w451 w470 w503 w529 w544 w568 w591 w609 w627 w644 w657 w674 w687 w706 w721 w740 w763 w785 w797 w817 w825] -> w440
            tunnel: w446 -> [w449 w468 w488 w515 w539 w558 w580 w599 w617 w635 w655 w669 w683 w700 w715 w730 w754 w773 w792 w811 w821 w826]
            tunnel: w447 -> [_ w467 w487 w514 w538 w557 w579 w598 w616 w634 w654 w668 w684 w701 w716 w731 w753 w772 w793 w810 w822 w827]
            tunnel: ["INVALID_PARAMETER" "DONE" "DONE" "DONE" "DONE" "DONE" "DONE" "DONE" "DONE" "DONE" "DONE" "DONE" "DONE" "DONE" "DONE" "DONE" "DONE" "DONE" "DONE" "DONE" "DONE" "DONE"] -> w439
            frame "False", Default {
            }
            frame "EXPTIME" {
              n179 = call "Read Tx Value.vi"("error in (no error)"=w468, "RxTx in"=w467) -> ("error out"=w458:errorcluster, "Rx Value"=w466:string)  [unwired: 7 in, 1 out]
              n180 = Unbundle By Name(w463) -> ("Simulated_Image_Constructor.lvclass"=w459:refnum<class "Simulated_Image_Constructor.lvclass">)
              n181 = Fract/Exp String To Number(string=w466, default (0 dbl)=sgl 0.0) -> (number=w469:sgl)  [unwired: 2 in, 1 out]
              n182 = call "Read Simulated_CCD_Camera.lvclass.vi"("error in (no error)"=w458, "Image Constructor in"=w459) -> ("error out"=w457:errorcluster, "Simulated_CCD_Camera.lvclass"=w456:refnum<class "Simulated_CCD_Camera.lvclass">, "Image Constructor out"=w454:refnum<class "Simulated_Image_Constructor.lvclass">)  [unwired: 7 in]
              n183 = call "Write Exposure Time.vi"("error in (no error)"=w457, "Exposure Time"=w469, "CCDCamera in"=w456) -> ("error out"=w464:errorcluster, "CCDCamera out"=w465:refnum<class "Simulated_CCD_Camera.lvclass">)  [unwired: 7 in]
              n184 = call-dynamic "Set Exposure Time.vi"("error in (no error)"=w464, "CCDCamera in"=w465) -> ("error out"=w453:errorcluster, "CCDCamera out"=w452:refnum<class "Simulated_CCD_Camera.lvclass">)  [unwired: 8 in]
              n185 = call "Write Simulated_CCD_Camera.lvclass.vi"("error in (no error)"=w453, "Simulated_CCD_Camera.lvclass"=w452, "Image Constructor in"=w454) -> ("error out"=w451:errorcluster, "Image Constructor out"=w455:refnum<class "Simulated_Image_Constructor.lvclass">)  [unwired: 7 in]
              n186 = Bundle By Name(cluster=w463, "Simulated_Image_Constructor.lvclass"=w455) -> (w462:refnum<class "Channel.lvclass">)
            }
            frame "READOUT" {
              n187 = call "Read Tx Value.vi"("error in (no error)"=w488, "RxTx in"=w487) -> ("error out"=w477:errorcluster, "Rx Value"=w483:string)  [unwired: 7 in, 1 out]
              n188 = Unbundle By Name(w489) -> ("Simulated_Image_Constructor.lvclass"=w478:refnum<class "Simulated_Image_Constructor.lvclass">)
              n189 = call "Read Simulated_CCD_Camera.lvclass.vi"("error in (no error)"=w477, "Image Constructor in"=w478) -> ("error out"=w475:errorcluster, "Simulated_CCD_Camera.lvclass"=w476:refnum<class "Simulated_CCD_Camera.lvclass">, "Image Constructor out"=w472:refnum<class "Simulated_Image_Constructor.lvclass">)  [unwired: 7 in]
              n190 = call "Read EM Mode.vi"("error in (no error)"=w475, "CCDCamera in"=w476) -> ("error out"=w481:errorcluster, "EM Mode"=w484:u8, "CCDCamera out"=w480:refnum<class "Simulated_CCD_Camera.lvclass">)  [unwired: 7 in]
              n191 = case shown="1" w484 {
                tunnel: w483 -> [w492 w496]
                tunnel: [w491 w495] -> w482
                frame 0, Default {
                  n192 = case shown="\"0.1\"" w492 {
                    tunnel: [_ 0 1] -> w491
                    frame "False", Default {
                    }
                    frame "0.1" {
                    }
                    frame "1" {
                    }
                  }
                }
                frame 1 {
                  n193 = case shown="\"30\"" w496 {
                    tunnel: [_ 0 1 2 3] -> w495
                    frame "False", Default {
                    }
                    frame "30" {
                    }
                    frame "20" {
                    }
                    frame "10" {
                    }
                    frame "1" {
                    }
                  }
                }
              }
              n194 = call "Write Readout Rate.vi"("error in (no error)"=w481, "Readout Rate"=w482, "CCDCamera in"=w480) -> ("error out"=w485:errorcluster, "CCDCamera out"=w486:refnum<class "Simulated_CCD_Camera.lvclass">)  [unwired: 7 in]
              n195 = call-dynamic "Set HSS and EM Mode.vi"("error in (no error)"=w485, "CCDCamera in"=w486) -> ("error out"=w473:errorcluster, "CCDCamera out"=w474:refnum<class "Simulated_CCD_Camera.lvclass">)  [unwired: 8 in]
              n196 = call "Write Simulated_CCD_Camera.lvclass.vi"("error in (no error)"=w473, "Simulated_CCD_Camera.lvclass"=w474, "Image Constructor in"=w472) -> ("error out"=w470:errorcluster, "Image Constructor out"=w471:refnum<class "Simulated_Image_Constructor.lvclass">)  [unwired: 7 in]
              n197 = Bundle By Name(cluster=w489, "Simulated_Image_Constructor.lvclass"=w471) -> (w490:refnum<class "Channel.lvclass">)
            }
            frame "BINNING" {
              n198 = call "Read Tx Value.vi"("error in (no error)"=w515, "RxTx in"=w514) -> ("error out"=w508:errorcluster, "Rx Value"=w513:string)  [unwired: 7 in, 1 out]
              n199 = Unbundle By Name(w517) -> ("Simulated_Image_Constructor.lvclass"=w509:refnum<class "Simulated_Image_Constructor.lvclass">)
              n200 = Decimal String To Number(string=w513) -> (number=w516:i32)  [unwired: 2 in, 1 out]
              n201 = call "Read Simulated_CCD_Camera.lvclass.vi"("error in (no error)"=w508, "Image Constructor in"=w509) -> ("error out"=w507:errorcluster, "Simulated_CCD_Camera.lvclass"=w506:refnum<class "Simulated_CCD_Camera.lvclass">, "Image Constructor out"=w501:refnum<class "Simulated_Image_Constructor.lvclass">)  [unwired: 7 in]
              n202 = call "Write Binning.vi"("error in (no error)"=w507, "Binning"=w516, "CCDCamera in"=w506) -> ("error out"=w511:errorcluster, "CCDCamera out"=w512:refnum<class "Simulated_CCD_Camera.lvclass">)  [unwired: 7 in]
              n203 = call-dynamic "Set Image.vi"("error in (no error)"=w511, "CCDCamera in"=w512) -> ("error out"=w504:errorcluster, "CCDCamera out"=w505:refnum<class "Simulated_CCD_Camera.lvclass">)  [unwired: 8 in]
              n204 = call "Write Simulated_CCD_Camera.lvclass.vi"("error in (no error)"=w504, "Simulated_CCD_Camera.lvclass"=w505, "Image Constructor in"=w501) -> ("error out"=w503:errorcluster, "Image Constructor out"=w502:refnum<class "Simulated_Image_Constructor.lvclass">)  [unwired: 7 in]
              n205 = Bundle By Name(cluster=w517, "Simulated_Image_Constructor.lvclass"=w502) -> (w518:refnum<class "Channel.lvclass">)
            }
            frame "COOLER" {
              n206 = call "Read Tx Value.vi"("error in (no error)"=w539, "RxTx in"=w538) -> ("error out"=w523:errorcluster, "Rx Value"=w534:string)  [unwired: 7 in, 1 out]
              n207 = Unbundle By Name(w540) -> ("Simulated_Image_Constructor.lvclass"=w527:refnum<class "Simulated_Image_Constructor.lvclass">)
              n208 = call "Read Simulated_CCD_Camera.lvclass.vi"("error in (no error)"=w523, "Image Constructor in"=w527) -> ("error out"=w524:errorcluster, "Simulated_CCD_Camera.lvclass"=w525:refnum<class "Simulated_CCD_Camera.lvclass">, "Image Constructor out"=w526:refnum<class "Simulated_Image_Constructor.lvclass">)  [unwired: 7 in]
              n209 = case shown="\"OFFe\", Default" w534 {
                tunnel: [0 1] -> w533
                frame "OFFe", Default {
                }
                frame "ON" {
                }
              }
              n210 = call-dynamic "Read Cooler.lvclass.vi"("error in (no error)"=w524, "CCDCamera in"=w525) -> ("error out"=w536:errorcluster, "Simulated_Cooler.lvclass"=w537:refnum<class "Simulated_Cooler.lvclass">, "CCDCamera out"=w535:refnum<class "Simulated_CCD_Camera.lvclass">)  [unwired: 7 in]
              n211 = call "Write Cooler ON_OFF.vi"("error in (no error)"=w536, "Cooler ON/OFF"=w533, "Cooler in"=w537) -> ("error out"=w519:errorcluster, "Cooler out"=w522:refnum<class "Simulated_Cooler.lvclass">)  [unwired: 7 in]
              n212 = call-dynamic "Set Cooler ON - OFF.vi"("error in (no error)"=w519, "Cooler in"=w522) -> ("error out"=w520:errorcluster, "Cooler out"=w521:refnum<class "Simulated_Cooler.lvclass">)  [unwired: 8 in]
              n213 = call-dynamic "Write Cooler.lvclass.vi"("error in (no error)"=w520, "Simulated_Cooler.lvclass"=w521, "CCDCamera in"=w535) -> ("error out"=w530:errorcluster, "CCDCamera out"=w531:refnum<class "Simulated_CCD_Camera.lvclass">)  [unwired: 7 in]
              n214 = call "Write Simulated_CCD_Camera.lvclass.vi"("error in (no error)"=w530, "Simulated_CCD_Camera.lvclass"=w531, "Image Constructor in"=w526) -> ("error out"=w529:errorcluster, "Image Constructor out"=w528:refnum<class "Simulated_Image_Constructor.lvclass">)  [unwired: 7 in]
              n215 = Bundle By Name(cluster=w540, "Simulated_Image_Constructor.lvclass"=w528) -> (w541:refnum<class "Channel.lvclass">)
            }
            frame "EM_GAIN" {
              n216 = call "Read Tx Value.vi"("error in (no error)"=w558, "RxTx in"=w557) -> ("error out"=w551:errorcluster, "Rx Value"=w556:string)  [unwired: 7 in, 1 out]
              n217 = Unbundle By Name(w560) -> ("Simulated_Image_Constructor.lvclass"=w552:refnum<class "Simulated_Image_Constructor.lvclass">)
              n218 = Decimal String To Number(string=w556) -> (number=w559:i32)  [unwired: 2 in, 1 out]
              n219 = call "Read Simulated_CCD_Camera.lvclass.vi"("error in (no error)"=w551, "Image Constructor in"=w552) -> ("error out"=w550:errorcluster, "Simulated_CCD_Camera.lvclass"=w549:refnum<class "Simulated_CCD_Camera.lvclass">, "Image Constructor out"=w546:refnum<class "Simulated_Image_Constructor.lvclass">)  [unwired: 7 in]
              n220 = call "Write EM Gain.vi"("error in (no error)"=w550, "EM Gain"=w559, "CCDCamera in"=w549) -> ("error out"=w555:errorcluster, "CCDCamera out"=w554:refnum<class "Simulated_CCD_Camera.lvclass">)  [unwired: 7 in]
              n221 = call-dynamic "Set EM Gain.vi"("error in (no error)"=w555, "CCDCamera in"=w554) -> ("error out"=w547:errorcluster, "CCDCamera out"=w548:refnum<class "Simulated_CCD_Camera.lvclass">)  [unwired: 8 in]
              n222 = call "Write Simulated_CCD_Camera.lvclass.vi"("error in (no error)"=w547, "Simulated_CCD_Camera.lvclass"=w548, "Image Constructor in"=w546) -> ("error out"=w544:errorcluster, "Image Constructor out"=w545:refnum<class "Simulated_Image_Constructor.lvclass">)  [unwired: 7 in]
              n223 = Bundle By Name(cluster=w560, "Simulated_Image_Constructor.lvclass"=w545) -> (w561:refnum<class "Channel.lvclass">)
            }
            frame "EM_MODE" {
              n224 = call "Read Tx Value.vi"("error in (no error)"=w580, "RxTx in"=w579) -> ("error out"=w565:errorcluster, "Rx Value"=w578:string)  [unwired: 7 in, 1 out]
              n225 = Unbundle By Name(w581) -> ("Simulated_Image_Constructor.lvclass"=w566:refnum<class "Simulated_Image_Constructor.lvclass">)
              n226 = case shown="\"EM\"" w578 {
                tunnel: [1 0] -> w577
                frame "CONVENTIONAL", Default {
                }
                frame "EM" {
                }
              }
              n227 = call "Read Simulated_CCD_Camera.lvclass.vi"("error in (no error)"=w565, "Image Constructor in"=w566) -> ("error out"=w564:errorcluster, "Simulated_CCD_Camera.lvclass"=w563:refnum<class "Simulated_CCD_Camera.lvclass">, "Image Constructor out"=w562:refnum<class "Simulated_Image_Constructor.lvclass">)  [unwired: 7 in]
              n228 = call "Write EM Mode.vi"("error in (no error)"=w564, "EM Mode"=w577, "CCDCamera in"=w563) -> ("error out"=w573:errorcluster, "CCDCamera out"=w576:refnum<class "Simulated_CCD_Camera.lvclass">)  [unwired: 7 in]
              n229 = call "Write Readout Rate.vi"("error in (no error)"=w573, "Readout Rate"=0, "CCDCamera in"=w576) -> ("error out"=w574:errorcluster, "CCDCamera out"=w575:refnum<class "Simulated_CCD_Camera.lvclass">)  [unwired: 7 in]
              n230 = call-dynamic "Set HSS and EM Mode.vi"("error in (no error)"=w574, "CCDCamera in"=w575) -> ("error out"=w567:errorcluster, "CCDCamera out"=w570:refnum<class "Simulated_CCD_Camera.lvclass">)  [unwired: 8 in]
              n231 = call "Write Simulated_CCD_Camera.lvclass.vi"("error in (no error)"=w567, "Simulated_CCD_Camera.lvclass"=w570, "Image Constructor in"=w562) -> ("error out"=w568:errorcluster, "Image Constructor out"=w569:refnum<class "Simulated_Image_Constructor.lvclass">)  [unwired: 7 in]
              n232 = Bundle By Name(cluster=w581, "Simulated_Image_Constructor.lvclass"=w569) -> (w582:refnum<class "Channel.lvclass">)
            }
            frame "FINAL_COLUMN" {
              n233 = call "Read Tx Value.vi"("error in (no error)"=w599, "RxTx in"=w598) -> ("error out"=w588:errorcluster, "Rx Value"=w597:string)  [unwired: 7 in, 1 out]
              n234 = Unbundle By Name(w601) -> ("Simulated_Image_Constructor.lvclass"=w589:refnum<class "Simulated_Image_Constructor.lvclass">)
              n235 = Decimal String To Number(string=w597) -> (number=w600:i32)  [unwired: 2 in, 1 out]
              n236 = call "Read Simulated_CCD_Camera.lvclass.vi"("error in (no error)"=w588, "Image Constructor in"=w589) -> ("error out"=w587:errorcluster, "Simulated_CCD_Camera.lvclass"=w586:refnum<class "Simulated_CCD_Camera.lvclass">, "Image Constructor out"=w585:refnum<class "Simulated_Image_Constructor.lvclass">)  [unwired: 7 in]
              n237 = call "Write Final Column.vi"("error in (no error)"=w587, "Final Column"=w600, "CCDCamera in"=w586) -> ("error out"=w595:errorcluster, "CCDCamera out"=w596:refnum<class "Simulated_CCD_Camera.lvclass">)  [unwired: 7 in]
              n238 = call-dynamic "Set Image.vi"("error in (no error)"=w595, "CCDCamera in"=w596) -> ("error out"=w592:errorcluster, "CCDCamera out"=w593:refnum<class "Simulated_CCD_Camera.lvclass">)  [unwired: 8 in]
              n239 = call "Write Simulated_CCD_Camera.lvclass.vi"("error in (no error)"=w592, "Simulated_CCD_Camera.lvclass"=w593, "Image Constructor in"=w585) -> ("error out"=w591:errorcluster, "Image Constructor out"=w590:refnum<class "Simulated_Image_Constructor.lvclass">)  [unwired: 7 in]
              n240 = Bundle By Name(cluster=w601, "Simulated_Image_Constructor.lvclass"=w590) -> (w602:refnum<class "Channel.lvclass">)
            }
            frame "FINAL_LINE" {
              n241 = Unbundle By Name(w619) -> ("Simulated_Image_Constructor.lvclass"=w607:refnum<class "Simulated_Image_Constructor.lvclass">)
              n242 = call "Read Tx Value.vi"("error in (no error)"=w617, "RxTx in"=w616) -> ("error out"=w603:errorcluster, "Rx Value"=w615:string)  [unwired: 7 in, 1 out]
              n243 = Decimal String To Number(string=w615) -> (number=w618:i32)  [unwired: 2 in, 1 out]
              n244 = call "Read Simulated_CCD_Camera.lvclass.vi"("error in (no error)"=w603, "Image Constructor in"=w607) -> ("error out"=w604:errorcluster, "Simulated_CCD_Camera.lvclass"=w605:refnum<class "Simulated_CCD_Camera.lvclass">, "Image Constructor out"=w606:refnum<class "Simulated_Image_Constructor.lvclass">)  [unwired: 7 in]
              n245 = call "Write Final Line.vi"("error in (no error)"=w604, "Final Line"=w618, "CCDCamera in"=w605) -> ("error out"=w613:errorcluster, "CCDCamera out"=w614:refnum<class "Simulated_CCD_Camera.lvclass">)  [unwired: 7 in]
              n246 = call-dynamic "Set Image.vi"("error in (no error)"=w613, "CCDCamera in"=w614) -> ("error out"=w610:errorcluster, "CCDCamera out"=w611:refnum<class "Simulated_CCD_Camera.lvclass">)  [unwired: 8 in]
              n247 = call "Write Simulated_CCD_Camera.lvclass.vi"("error in (no error)"=w610, "Simulated_CCD_Camera.lvclass"=w611, "Image Constructor in"=w606) -> ("error out"=w609:errorcluster, "Image Constructor out"=w608:refnum<class "Simulated_Image_Constructor.lvclass">)  [unwired: 7 in]
              n248 = Bundle By Name(cluster=w619, "Simulated_Image_Constructor.lvclass"=w608) -> (w620:refnum<class "Channel.lvclass">)
            }
            frame "INITIAL_COLUMN" {
              n249 = Unbundle By Name(w637) -> ("Simulated_Image_Constructor.lvclass"=w625:refnum<class "Simulated_Image_Constructor.lvclass">)
              n250 = call "Read Tx Value.vi"("error in (no error)"=w635, "RxTx in"=w634) -> ("error out"=w622:errorcluster, "Rx Value"=w633:string)  [unwired: 7 in, 1 out]
              n251 = Decimal String To Number(string=w633) -> (number=w636:i32)  [unwired: 2 in, 1 out]
              n252 = call "Read Simulated_CCD_Camera.lvclass.vi"("error in (no error)"=w622, "Image Constructor in"=w625) -> ("error out"=w623:errorcluster, "Simulated_CCD_Camera.lvclass"=w621:refnum<class "Simulated_CCD_Camera.lvclass">, "Image Constructor out"=w624:refnum<class "Simulated_Image_Constructor.lvclass">)  [unwired: 7 in]
              n253 = call "Write Initial Cloumn.vi"("error in (no error)"=w623, "Initial Cloumn"=w636, "CCDCamera in"=w621) -> ("error out"=w631:errorcluster, "CCDCamera out"=w632:refnum<class "Simulated_CCD_Camera.lvclass">)  [unwired: 7 in]
              n254 = call-dynamic "Set Image.vi"("error in (no error)"=w631, "CCDCamera in"=w632) -> ("error out"=w628:errorcluster, "CCDCamera out"=w629:refnum<class "Simulated_CCD_Camera.lvclass">)  [unwired: 8 in]
              n255 = call "Write Simulated_CCD_Camera.lvclass.vi"("error in (no error)"=w628, "Simulated_CCD_Camera.lvclass"=w629, "Image Constructor in"=w624) -> ("error out"=w627:errorcluster, "Image Constructor out"=w626:refnum<class "Simulated_Image_Constructor.lvclass">)  [unwired: 7 in]
              n256 = Bundle By Name(cluster=w637, "Simulated_Image_Constructor.lvclass"=w626) -> (w638:refnum<class "Channel.lvclass">)
            }
            frame "INITIAL_LINE" {
              n257 = Unbundle By Name(w650) -> ("Simulated_Image_Constructor.lvclass"=w643:refnum<class "Simulated_Image_Constructor.lvclass">)
              n258 = call "Read Tx Value.vi"("error in (no error)"=w655, "RxTx in"=w654) -> ("error out"=w639:errorcluster, "Rx Value"=w653:string)  [unwired: 7 in, 1 out]
              n259 = Decimal String To Number(string=w653) -> (number=w656:i32)  [unwired: 2 in, 1 out]
              n260 = call "Read Simulated_CCD_Camera.lvclass.vi"("error in (no error)"=w639, "Image Constructor in"=w643) -> ("error out"=w640:errorcluster, "Simulated_CCD_Camera.lvclass"=w641:refnum<class "Simulated_CCD_Camera.lvclass">, "Image Constructor out"=w642:refnum<class "Simulated_Image_Constructor.lvclass">)  [unwired: 7 in]
              n261 = call "Write Initial Line.vi"("error in (no error)"=w640, "Initial Line"=w656, "CCDCamera in"=w641) -> ("error out"=w651:errorcluster, "CCDCamera out"=w652:refnum<class "Simulated_CCD_Camera.lvclass">)  [unwired: 7 in]
              n262 = call-dynamic "Set Image.vi"("error in (no error)"=w651, "CCDCamera in"=w652) -> ("error out"=w646:errorcluster, "CCDCamera out"=w647:refnum<class "Simulated_CCD_Camera.lvclass">)  [unwired: 8 in]
              n263 = call "Write Simulated_CCD_Camera.lvclass.vi"("error in (no error)"=w646, "Simulated_CCD_Camera.lvclass"=w647, "Image Constructor in"=w642) -> ("error out"=w644:errorcluster, "Image Constructor out"=w645:refnum<class "Simulated_Image_Constructor.lvclass">)  [unwired: 7 in]
              n264 = Bundle By Name(cluster=w650, "Simulated_Image_Constructor.lvclass"=w645) -> (w649:refnum<class "Channel.lvclass">)
            }
            frame "IMAGE_PATH" {
              n265 = call "Read Tx Value.vi"("error in (no error)"=w669, "RxTx in"=w668) -> ("error out"=w659:errorcluster, "Rx Value"=w667:string)  [unwired: 7 in, 1 out]
              n266 = Unbundle By Name(w670) -> ("Simulated_Image_Constructor.lvclass"=w660:refnum<class "Simulated_Image_Constructor.lvclass">)
              n267 = call "Read Save Image.lvclass.vi"("error in (no error)"=w659, "Image Constructor in"=w660) -> ("error out"=w662:errorcluster, "Save Image.lvclass"=w663:refnum<class "Save Image.lvclass">, "Image Constructor out"=w661:refnum<class "Simulated_Image_Constructor.lvclass">)  [unwired: 7 in]
              n268 = call "Write Image Path.vi"("error in (no error)"=w662, "Image Path"=w667, "Save Image in"=w663) -> ("error out"=w664:errorcluster, "Save Image out"=w665:refnum<class "Save Image.lvclass">)  [unwired: 7 in]
              n269 = call "Write Save Image.lvclass.vi"("error in (no error)"=w664, "Save Image.lvclass"=w665, "Image Constructor in"=w661) -> ("error out"=w657:errorcluster, "Image Constructor out"=w658:refnum<class "Simulated_Image_Constructor.lvclass">)  [unwired: 7 in]
              n270 = Bundle By Name(cluster=w670, "Simulated_Image_Constructor.lvclass"=w658) -> (w671:refnum<class "Channel.lvclass">)
            }
            frame "FILE_BASE_NAME" {
              n271 = Unbundle By Name(w685) -> ("Simulated_Image_Constructor.lvclass"=w672:refnum<class "Simulated_Image_Constructor.lvclass">)
              n272 = call "Read Tx Value.vi"("error in (no error)"=w683, "RxTx in"=w684) -> ("error out"=w673:errorcluster, "Rx Value"=w682:string)  [unwired: 7 in, 1 out]
              n273 = call "Read Save Image.lvclass.vi"("error in (no error)"=w673, "Image Constructor in"=w672) -> ("error out"=w677:errorcluster, "Save Image.lvclass"=w678:refnum<class "Save Image.lvclass">, "Image Constructor out"=w676:refnum<class "Simulated_Image_Constructor.lvclass">)  [unwired: 7 in]
              n274 = call "Write Image Base Name.vi"("error in (no error)"=w677, "Base Name"=w682, "Save Image in"=w678) -> ("error out"=w679:errorcluster, "Save Image out"=w680:refnum<class "Save Image.lvclass">)  [unwired: 7 in]
              n275 = call "Write Save Image.lvclass.vi"("error in (no error)"=w679, "Save Image.lvclass"=w680, "Image Constructor in"=w676) -> ("error out"=w674:errorcluster, "Image Constructor out"=w675:refnum<class "Simulated_Image_Constructor.lvclass">)  [unwired: 7 in]
              n276 = Bundle By Name(cluster=w685, "Simulated_Image_Constructor.lvclass"=w675) -> (w686:refnum<class "Channel.lvclass">)
            }
            frame "#INDEX" {
              # "This parameter does not exist anymore"
              n277 = Unbundle By Name(w702) -> ("Simulated_Image_Constructor.lvclass"=w690:refnum<class "Simulated_Image_Constructor.lvclass">)
              n278 = call "Read Tx Value.vi"("error in (no error)"=w700, "RxTx in"=w701) -> ("error out"=w689:errorcluster, "Rx Value"=w698:string)  [unwired: 7 in, 1 out]
              n279 = Decimal String To Number(string=w698, default (0L)=u16 0) -> (number=w697:u16)  [unwired: 1 in, 1 out]
              n280 = call "Read Save Image.lvclass.vi"("error in (no error)"=w689, "Image Constructor in"=w690) -> ("error out"=w692:errorcluster, "Save Image.lvclass"=w693:refnum<class "Save Image.lvclass">, "Image Constructor out"=w691:refnum<class "Simulated_Image_Constructor.lvclass">)  [unwired: 7 in]
              n281 = call "Write Image Index.vi"("error in (no error)"=w692, "Image Index"=w697, "Save Image in"=w693) -> ("error out"=w694:errorcluster, "Save Image out"=w695:refnum<class "Save Image.lvclass">)  [unwired: 7 in]
              n282 = call "Write Save Image.lvclass.vi"("error in (no error)"=w694, "Save Image.lvclass"=w695, "Image Constructor in"=w691) -> ("error out"=w687:errorcluster, "Image Constructor out"=w688:refnum<class "Simulated_Image_Constructor.lvclass">)  [unwired: 7 in]
              n283 = Bundle By Name(cluster=w702, "Simulated_Image_Constructor.lvclass"=w688) -> (w703:refnum<class "Channel.lvclass">)
            }
            frame "OBSERVATION_TITLE" {
              n284 = call "Read Tx Value.vi"("error in (no error)"=w715, "RxTx in"=w716) -> ("error out"=w705:errorcluster, "Rx Value"=w714:string)  [unwired: 7 in, 1 out]
              n285 = Unbundle By Name(w717) -> ("Simulated_Image_Constructor.lvclass"=w704:refnum<class "Simulated_Image_Constructor.lvclass">)
              n286 = call "Read Save Image.lvclass.vi"("error in (no error)"=w705, "Image Constructor in"=w704) -> ("error out"=w709:errorcluster, "Save Image.lvclass"=w710:refnum<class "Save Image.lvclass">, "Image Constructor out"=w708:refnum<class "Simulated_Image_Constructor.lvclass">)  [unwired: 7 in]
              n287 = call "Write Observation Title.vi"("error in (no error)"=w709, "OBS_TITLE.Value"=w714, "Save Image in"=w710) -> ("error out"=w711:errorcluster, "Save Image out"=w712:refnum<class "Save Image.lvclass">)  [unwired: 7 in]
              n288 = call "Write Save Image.lvclass.vi"("error in (no error)"=w711, "Save Image.lvclass"=w712, "Image Constructor in"=w708) -> ("error out"=w706:errorcluster, "Image Constructor out"=w707:refnum<class "Simulated_Image_Constructor.lvclass">)  [unwired: 7 in]
              n289 = Bundle By Name(cluster=w717, "Simulated_Image_Constructor.lvclass"=w707) -> (w718:refnum<class "Channel.lvclass">)
            }
            frame "COMMENT" {
              n290 = call "Read Tx Value.vi"("error in (no error)"=w730, "RxTx in"=w731) -> ("error out"=w720:errorcluster, "Rx Value"=w729:string)  [unwired: 7 in, 1 out]
              n291 = Unbundle By Name(w732) -> ("Simulated_Image_Constructor.lvclass"=w719:refnum<class "Simulated_Image_Constructor.lvclass">)
              n292 = call "Read Save Image.lvclass.vi"("error in (no error)"=w720, "Image Constructor in"=w719) -> ("error out"=w724:errorcluster, "Save Image.lvclass"=w725:refnum<class "Save Image.lvclass">, "Image Constructor out"=w723:refnum<class "Simulated_Image_Constructor.lvclass">)  [unwired: 7 in]
              n293 = call "Write Comment.vi"("error in (no error)"=w724, "COMMENT.Value"=w729, "Save Image in"=w725) -> ("error out"=w726:errorcluster, "Save Image out"=w727:refnum<class "Save Image.lvclass">)  [unwired: 7 in]
              n294 = call "Write Save Image.lvclass.vi"("error in (no error)"=w726, "Save Image.lvclass"=w727, "Image Constructor in"=w723) -> ("error out"=w721:errorcluster, "Image Constructor out"=w722:refnum<class "Simulated_Image_Constructor.lvclass">)  [unwired: 7 in]
              n295 = Bundle By Name(cluster=w732, "Simulated_Image_Constructor.lvclass"=w722) -> (w733:refnum<class "Channel.lvclass">)
            }
            frame "TEMPERATURE" {
              n296 = Unbundle By Name(w755) -> ("Simulated_Image_Constructor.lvclass"=w735:refnum<class "Simulated_Image_Constructor.lvclass">)
              n297 = call "Read Tx Value.vi"("error in (no error)"=w754, "RxTx in"=w753) -> ("error out"=w734:errorcluster, "Rx Value"=w752:string)  [unwired: 7 in, 1 out]
              n298 = Decimal String To Number(string=w752) -> (number=w745:i32)  [unwired: 2 in, 1 out]
              n299 = call "Read Simulated_CCD_Camera.lvclass.vi"("error in (no error)"=w734, "Image Constructor in"=w735) -> ("error out"=w738:errorcluster, "Simulated_CCD_Camera.lvclass"=w737:refnum<class "Simulated_CCD_Camera.lvclass">, "Image Constructor out"=w736:refnum<class "Simulated_Image_Constructor.lvclass">)  [unwired: 7 in]
              n300 = call-dynamic "Read Cooler.lvclass.vi"("error in (no error)"=w738, "CCDCamera in"=w737) -> ("error out"=w750:errorcluster, "Simulated_Cooler.lvclass"=w751:refnum<class "Simulated_Cooler.lvclass">, "CCDCamera out"=w744:refnum<class "Simulated_CCD_Camera.lvclass">)  [unwired: 7 in]
              n301 = call-dynamic "Write Temperature.vi"("error in (no error)"=w750, "Temperature"=w745, "Cooler in"=w751) -> ("error out"=w746:errorcluster, "Cooler out"=w747:refnum<class "Simulated_Cooler.lvclass">)  [unwired: 7 in]
              n302 = call-dynamic "Set Temperature.vi"("error in (no error)"=w746, "Cooler in"=w747) -> ("error out"=w748:errorcluster, "Cooler out"=w749:refnum<class "Simulated_Cooler.lvclass">)  [unwired: 8 in]
              n303 = call-dynamic "Write Cooler.lvclass.vi"("error in (no error)"=w748, "Simulated_Cooler.lvclass"=w749, "CCDCamera in"=w744) -> ("error out"=w741:errorcluster, "CCDCamera out"=w742:refnum<class "Simulated_CCD_Camera.lvclass">)  [unwired: 7 in]
              n304 = call "Write Simulated_CCD_Camera.lvclass.vi"("error in (no error)"=w741, "Simulated_CCD_Camera.lvclass"=w742, "Image Constructor in"=w736) -> ("error out"=w740:errorcluster, "Image Constructor out"=w739:refnum<class "Simulated_Image_Constructor.lvclass">)  [unwired: 7 in]
              n305 = Bundle By Name(cluster=w755, "Simulated_Image_Constructor.lvclass"=w739) -> (w756:refnum<class "Channel.lvclass">)
            }
            frame "SHUTTER" {
              n306 = call "Read Tx Value.vi"("error in (no error)"=w773, "RxTx in"=w772) -> ("error out"=w757:errorcluster, "Rx Value"=w767:string)  [unwired: 7 in, 1 out]
              n307 = Unbundle By Name(w774) -> ("Simulated_Image_Constructor.lvclass"=w761:refnum<class "Simulated_Image_Constructor.lvclass">)
              n308 = To Upper Case(1:w767) -> (0:w768:string)
              n309 = case shown="\"OPEN\"" w768 {
                tunnel: [2 1 0] -> w769
                frame "CLOSED", Default {
                }
                frame "OPEN" {
                }
                frame "AUTO" {
                }
              }
              n310 = call "Read Simulated_CCD_Camera.lvclass.vi"("error in (no error)"=w757, "Image Constructor in"=w761) -> ("error out"=w758:errorcluster, "Simulated_CCD_Camera.lvclass"=w759:refnum<class "Simulated_CCD_Camera.lvclass">, "Image Constructor out"=w760:refnum<class "Simulated_Image_Constructor.lvclass">)  [unwired: 7 in]
              n311 = call "Write Shutter Mode.vi"("error in (no error)"=w758, "Shutter Mode"=w769, "CCDCamera in"=w759) -> ("error out"=w770:errorcluster, "CCDCamera out"=w771:refnum<class "Simulated_CCD_Camera.lvclass">)  [unwired: 7 in]
              n312 = call-dynamic "Set Shutter Mode.vi"("error in (no error)"=w770, "CCDCamera in"=w771) -> ("error out"=w764:errorcluster, "CCDCamera out"=w765:refnum<class "Simulated_CCD_Camera.lvclass">)  [unwired: 8 in]
              n313 = call "Write Simulated_CCD_Camera.lvclass.vi"("error in (no error)"=w764, "Simulated_CCD_Camera.lvclass"=w765, "Image Constructor in"=w760) -> ("error out"=w763:errorcluster, "Image Constructor out"=w762:refnum<class "Simulated_Image_Constructor.lvclass">)  [unwired: 7 in]
              n314 = Bundle By Name(cluster=w774, "Simulated_Image_Constructor.lvclass"=w762) -> (w775:refnum<class "Channel.lvclass">)
            }
            frame "PREAMP" {
              n315 = call "Read Tx Value.vi"("error in (no error)"=w792, "RxTx in"=w793) -> ("error out"=w782:errorcluster, "Rx Value"=w791:string)  [unwired: 7 in, 1 out]
              n316 = Unbundle By Name(w795) -> ("Simulated_Image_Constructor.lvclass"=w783:refnum<class "Simulated_Image_Constructor.lvclass">)
              n317 = Decimal String To Number(string=w791) -> (number=w794:i32)  [unwired: 2 in, 1 out]
              n318 = call "Read Simulated_CCD_Camera.lvclass.vi"("error in (no error)"=w782, "Image Constructor in"=w783) -> ("error out"=w781:errorcluster, "Simulated_CCD_Camera.lvclass"=w780:refnum<class "Simulated_CCD_Camera.lvclass">, "Image Constructor out"=w779:refnum<class "Simulated_Image_Constructor.lvclass">)  [unwired: 7 in]
              n319 = call "Write Pre-amp gain.vi"("error in (no error)"=w781, "Pre-amp gain"=w794, "CCDCamera in"=w780) -> ("error out"=w789:errorcluster, "CCDCamera out"=w790:refnum<class "Simulated_CCD_Camera.lvclass">)  [unwired: 7 in]
              n320 = call-dynamic "Set Pre Amplification.vi"("error in (no error)"=w789, "CCDCamera in"=w790) -> ("error out"=w786:errorcluster, "CCDCamera out"=w787:refnum<class "Simulated_CCD_Camera.lvclass">)  [unwired: 8 in]
              n321 = call "Write Simulated_CCD_Camera.lvclass.vi"("error in (no error)"=w786, "Simulated_CCD_Camera.lvclass"=w787, "Image Constructor in"=w779) -> ("error out"=w785:errorcluster, "Image Constructor out"=w784:refnum<class "Simulated_Image_Constructor.lvclass">)  [unwired: 7 in]
              n322 = Bundle By Name(cluster=w795, "Simulated_Image_Constructor.lvclass"=w784) -> (w796:refnum<class "Channel.lvclass">)
            }
            frame "KSERLEN" {
              n323 = call "Read Tx Value.vi"("error in (no error)"=w811, "RxTx in"=w810) -> ("error out"=w799:errorcluster, "Rx Value"=w809:string)  [unwired: 7 in, 1 out]
              n324 = Unbundle By Name(w813) -> ("Simulated_Image_Constructor.lvclass"=w803:refnum<class "Simulated_Image_Constructor.lvclass">)
              n325 = Decimal String To Number(string=w809) -> (number=w812:i32)  [unwired: 2 in, 1 out]
              n326 = call "Read Simulated_CCD_Camera.lvclass.vi"("error in (no error)"=w799, "Image Constructor in"=w803) -> ("error out"=w800:errorcluster, "Simulated_CCD_Camera.lvclass"=w801:refnum<class "Simulated_CCD_Camera.lvclass">, "Image Constructor out"=w802:refnum<class "Simulated_Image_Constructor.lvclass">)  [unwired: 7 in]
              n327 = call "Write Kinetic Series Length.vi"("error in (no error)"=w800, "Kinetic Series Length"=w812, "CCDCamera in"=w801) -> ("error out"=w807:errorcluster, "CCDCamera out"=w808:refnum<class "Simulated_CCD_Camera.lvclass">)  [unwired: 7 in]
              n328 = call-dynamic "Set Kinetic Series Length.vi"("error in (no error)"=w807, "CCDCamera in"=w808) -> ("error out"=w804:errorcluster, "CCDCamera out"=w805:refnum<class "Simulated_CCD_Camera.lvclass">)  [unwired: 8 in]
              n329 = call "Write Simulated_CCD_Camera.lvclass.vi"("error in (no error)"=w804, "Simulated_CCD_Camera.lvclass"=w805, "Image Constructor in"=w802) -> ("error out"=w797:errorcluster, "Image Constructor out"=w798:refnum<class "Simulated_Image_Constructor.lvclass">)  [unwired: 7 in]
              n330 = Bundle By Name(cluster=w813, "Simulated_Image_Constructor.lvclass"=w798) -> (w814:refnum<class "Channel.lvclass">)
            }
            frame "CUBES" {
              n331 = call "Read Tx Value.vi"("error in (no error)"=w821, "RxTx in"=w822) -> ("error out"=w817:errorcluster, "Rx Value"=w819:string)  [unwired: 7 in, 1 out]
              n332 = Decimal String To Number(string=w819) -> (number=w818:i32)  [unwired: 2 in, 1 out]
              n333 = Bundle By Name(cluster=w820, "Cubes"=w818) -> (w816:refnum<class "Channel.lvclass">)
            }
            frame "DS9" {
              # "This parameter is wrong"
              n334 = call "Read Tx Value.vi"("error in (no error)"=w826, "RxTx in"=w827) -> ("error out"=w825:errorcluster)  [unwired: 7 in, 2 out]
            }
          }
          n335 = Unbundle By Name(w443) -> ("RxTx.lvclass"=w442:refnum<class "RxTx.lvclass">)
          n336 = call "Send TX Message.vi"("error in (no error)"=w440, "element"=w439, "RxTx in"=w442) -> ("error out"=w433:errorcluster, "RxTx out"=w441:refnum<class "RxTx.lvclass">)  [unwired: 7 in]
          n337 = Bundle By Name(cluster=w443, "RxTx.lvclass"=w441) -> (w432:refnum<class "Channel.lvclass">)
          n338 = Unbundle By Name(w432) -> ("State Machine.lvclass"=w435:refnum<class "State Machine.lvclass">)
          n339 = call-dynamic "Write State.vi"("error in (no error)"=w433, "State"="False", "State Machine in"=w435) -> ("error out"=w430:errorcluster, "State Machine out"=w436:refnum<class "State Machine.lvclass">)  [unwired: 7 in]
          n340 = Bundle By Name(cluster=w432, "State Machine.lvclass"=w436) -> (w431:refnum<class "Channel.lvclass">)
        }
        frame "GET" {
          n341 = Unbundle By Name(w837) -> ("RxTx.lvclass"=w843:refnum<class "RxTx.lvclass">)
          n342 = call "Read Rx Value.vi"("error in (no error)"=w836, "RxTx in"=w843) -> ("error out"=w844:errorcluster, "Rx value"=w828:string)  [unwired: 7 in, 1 out]
          n343 = case shown="\"KSERLEN\"" w828 {
            tunnel: [w847 w855 w863 w871 w879 w885 w895 w903 w911 w919 w927 w935 w943 w951 w958 w965 w973 w981 w989 w997 w1001] -> w840
            tunnel: w837 -> [w847 w855 w863 w871 w879 w885 w895 w903 w911 w919 w927 w935 w943 w951 w958 w965 w973 w981 w989 w997 w1001]
            tunnel: [w846 w853 w861 w869 w877 w886 w893 w901 w909 w917 w925 w933 w942 w949 w957 w964 w971 w979 w987 w995 w999] -> w839
            tunnel: w844 -> [w846 w850 w858 w864 w874 w880 w890 w897 w904 w912 w920 w928 w936 w944 w952 w959 w966 w974 w982 w990 w999]
            tunnel: ["INVALID_PARAMETER" w852 w860 w868 w876 w884 w892 w900 w908 w916 w924 w932 w940 w948 w956 w963 w970 w978 w986 w994 w998] -> w838
            frame "False", Default {
            }
            frame "EXPTIME" {
              n344 = Unbundle By Name(w855) -> ("Simulated_Image_Constructor.lvclass"=w851:refnum<class "Simulated_Image_Constructor.lvclass">)
              n345 = call "Read Simulated_CCD_Camera.lvclass.vi"("error in (no error)"=w850, "Image Constructor in"=w851) -> ("error out"=w848:errorcluster, "Simulated_CCD_Camera.lvclass"=w849:refnum<class "Simulated_CCD_Camera.lvclass">)  [unwired: 7 in, 1 out]
              n346 = call "Read Exposure Time.vi"("error in (no error)"=w848, "CCDCamera in"=w849) -> ("error out"=w853:errorcluster, "Exposure Time"=w854:sgl)  [unwired: 7 in, 1 out]
              n347 = Number To Fractional String(number=w854) -> (F-format string=w852:string)  [unwired: 3 in]
            }
            frame "READOUT" {
              n348 = Unbundle By Name(w863) -> ("Simulated_Image_Constructor.lvclass"=w859:refnum<class "Simulated_Image_Constructor.lvclass">)
              n349 = call "Read Simulated_CCD_Camera.lvclass.vi"("error in (no error)"=w858, "Image Constructor in"=w859) -> ("error out"=w856:errorcluster, "Simulated_CCD_Camera.lvclass"=w857:refnum<class "Simulated_CCD_Camera.lvclass">)  [unwired: 7 in, 1 out]
              n350 = call "Read Readout Rate.vi"("error in (no error)"=w856, "CCDCamera in"=w857) -> ("error out"=w861:errorcluster, "Readout Rate"=w862:u8)  [unwired: 7 in, 1 out]
              n351 = Number To Decimal String(number=w862) -> (decimal integer string=w860:string)  [unwired: 1 in]
            }
            frame "BINNING" {
              n352 = Unbundle By Name(w871) -> ("Simulated_Image_Constructor.lvclass"=w865:refnum<class "Simulated_Image_Constructor.lvclass">)
              n353 = call "Read Simulated_CCD_Camera.lvclass.vi"("error in (no error)"=w864, "Image Constructor in"=w865) -> ("error out"=w867:errorcluster, "Simulated_CCD_Camera.lvclass"=w866:refnum<class "Simulated_CCD_Camera.lvclass">)  [unwired: 7 in, 1 out]
              n354 = call "Read Binning.vi"("error in (no error)"=w867, "CCDCamera in"=w866) -> ("error out"=w869:errorcluster, "Binning"=w870:u16)  [unwired: 7 in, 1 out]
              n355 = Number To Decimal String(number=w870) -> (decimal integer string=w868:string)  [unwired: 1 in]
            }
            frame "COOLER" {
              n356 = Unbundle By Name(w879) -> ("Simulated_Image_Constructor.lvclass"=w875:refnum<class "Simulated_Image_Constructor.lvclass">)
              n357 = call "Read Simulated_CCD_Camera.lvclass.vi"("error in (no error)"=w874, "Image Constructor in"=w875) -> ("error out"=w873:errorcluster, "Simulated_CCD_Camera.lvclass"=w872:refnum<class "Simulated_CCD_Camera.lvclass">)  [unwired: 7 in, 1 out]
              n358 = call "Read Cooler ON_OFF.vi"("error in (no error)"=w873, "CCDCamera in"=w872) -> ("error out"=w877:errorcluster, "Cooler ON/OFF"=w878:u8)  [unwired: 7 in, 1 out]
              n359 = Number To Decimal String(number=w878) -> (decimal integer string=w876:string)  [unwired: 1 in]
            }
            frame "EM_GAIN" {
              n360 = Unbundle By Name(w885) -> ("Simulated_Image_Constructor.lvclass"=w881:refnum<class "Simulated_Image_Constructor.lvclass">)
              n361 = call "Read Simulated_CCD_Camera.lvclass.vi"("error in (no error)"=w880, "Image Constructor in"=w881) -> ("error out"=w883:errorcluster, "Simulated_CCD_Camera.lvclass"=w882:refnum<class "Simulated_CCD_Camera.lvclass">)  [unwired: 7 in, 1 out]
              n362 = call "Read EM Gain.vi"("error in (no error)"=w883, "CCDCamera in"=w882) -> ("error out"=w886:errorcluster, "EM Gain"=w887:u16)  [unwired: 7 in, 1 out]
              n363 = Number To Decimal String(number=w887) -> (decimal integer string=w884:string)  [unwired: 1 in]
            }
            frame "EM_MODE" {
              n364 = Unbundle By Name(w895) -> ("Simulated_Image_Constructor.lvclass"=w891:refnum<class "Simulated_Image_Constructor.lvclass">)
              n365 = call "Read Simulated_CCD_Camera.lvclass.vi"("error in (no error)"=w890, "Image Constructor in"=w891) -> ("error out"=w888:errorcluster, "Simulated_CCD_Camera.lvclass"=w889:refnum<class "Simulated_CCD_Camera.lvclass">)  [unwired: 7 in, 1 out]
              n366 = call "Read EM Mode.vi"("error in (no error)"=w888, "CCDCamera in"=w889) -> ("error out"=w893:errorcluster, "EM Mode"=w894:u8)  [unwired: 7 in, 1 out]
              n367 = Number To Decimal String(number=w894) -> (decimal integer string=w892:string)  [unwired: 1 in]
            }
            frame "FINAL_COLUMN" {
              n368 = Unbundle By Name(w903) -> ("Simulated_Image_Constructor.lvclass"=w896:refnum<class "Simulated_Image_Constructor.lvclass">)
              n369 = call "Read Simulated_CCD_Camera.lvclass.vi"("error in (no error)"=w897, "Image Constructor in"=w896) -> ("error out"=w898:errorcluster, "Simulated_CCD_Camera.lvclass"=w899:refnum<class "Simulated_CCD_Camera.lvclass">)  [unwired: 7 in, 1 out]
              n370 = call "Read Final Column.vi"("error in (no error)"=w898, "CCDCamera in"=w899) -> ("error out"=w901:errorcluster, "Final Column"=w902:u16)  [unwired: 7 in, 1 out]
              n371 = Number To Decimal String(number=w902) -> (decimal integer string=w900:string)  [unwired: 1 in]
            }
            frame "FINAL_LINE" {
              n372 = Unbundle By Name(w911) -> ("Simulated_Image_Constructor.lvclass"=w905:refnum<class "Simulated_Image_Constructor.lvclass">)
              n373 = call "Read Simulated_CCD_Camera.lvclass.vi"("error in (no error)"=w904, "Image Constructor in"=w905) -> ("error out"=w907:errorcluster, "Simulated_CCD_Camera.lvclass"=w906:refnum<class "Simulated_CCD_Camera.lvclass">)  [unwired: 7 in, 1 out]
              n374 = call "Read Final Line.vi"("error in (no error)"=w907, "CCDCamera in"=w906) -> ("error out"=w909:errorcluster, "Final Line"=w910:u16)  [unwired: 7 in, 1 out]
              n375 = Number To Decimal String(number=w910) -> (decimal integer string=w908:string)  [unwired: 1 in]
            }
            frame "INITIAL_COLUMN" {
              n376 = Unbundle By Name(w919) -> ("Simulated_Image_Constructor.lvclass"=w913:refnum<class "Simulated_Image_Constructor.lvclass">)
              n377 = call "Read Simulated_CCD_Camera.lvclass.vi"("error in (no error)"=w912, "Image Constructor in"=w913) -> ("error out"=w915:errorcluster, "Simulated_CCD_Camera.lvclass"=w914:refnum<class "Simulated_CCD_Camera.lvclass">)  [unwired: 7 in, 1 out]
              n378 = call "Read Initial Cloumn.vi"("error in (no error)"=w915, "CCDCamera in"=w914) -> ("error out"=w917:errorcluster, "Initial Cloumn"=w918:u16)  [unwired: 7 in, 1 out]
              n379 = Number To Decimal String(number=w918) -> (decimal integer string=w916:string)  [unwired: 1 in]
            }
            frame "INITIAL_LINE" {
              n380 = Unbundle By Name(w927) -> ("Simulated_Image_Constructor.lvclass"=w921:refnum<class "Simulated_Image_Constructor.lvclass">)
              n381 = call "Read Simulated_CCD_Camera.lvclass.vi"("error in (no error)"=w920, "Image Constructor in"=w921) -> ("error out"=w923:errorcluster, "Simulated_CCD_Camera.lvclass"=w922:refnum<class "Simulated_CCD_Camera.lvclass">)  [unwired: 7 in, 1 out]
              n382 = call "Read Initial Line.vi"("error in (no error)"=w923, "CCDCamera in"=w922) -> ("error out"=w925:errorcluster, "Initial Line"=w926:u16)  [unwired: 7 in, 1 out]
              n383 = Number To Decimal String(number=w926) -> (decimal integer string=w924:string)  [unwired: 1 in]
            }
            frame "IMAGE_PATH" {
              n384 = Unbundle By Name(w935) -> ("Simulated_Image_Constructor.lvclass"=w929:refnum<class "Simulated_Image_Constructor.lvclass">)
              n385 = call "Read Save Image.lvclass.vi"("error in (no error)"=w928, "Image Constructor in"=w929) -> ("error out"=w931:errorcluster, "Save Image.lvclass"=w930:refnum<class "Save Image.lvclass">)  [unwired: 7 in, 1 out]
              n386 = call "Read Image Information.vi"("error in (no error)"=w931, "Save Image in"=w930) -> ("error out"=w933:errorcluster, "Image Information"=w934:T6)  [unwired: 7 in, 1 out]
              n387 = Unbundle By Name(w934) -> ("Image Path"=w932:string)
            }
            frame "#INDEX" {
              n388 = Unbundle By Name(w943) -> ("Simulated_Image_Constructor.lvclass"=w937:refnum<class "Simulated_Image_Constructor.lvclass">)
              n389 = call "Read Save Image.lvclass.vi"("error in (no error)"=w936, "Image Constructor in"=w937) -> ("error out"=w939:errorcluster, "Save Image.lvclass"=w938:refnum<class "Save Image.lvclass">)  [unwired: 7 in, 1 out]
              n390 = call "Read Image Index.vi"("error in (no error)"=w939, "Save Image in"=w938) -> ("error out"=w942:errorcluster, "Image Index"=w941:u16)  [unwired: 7 in, 1 out]
              n391 = Number To Decimal String(number=w941) -> (decimal integer string=w940:string)  [unwired: 1 in]
            }
            frame "FILE_BASE_NAME" {
              n392 = Unbundle By Name(w951) -> ("Simulated_Image_Constructor.lvclass"=w945:refnum<class "Simulated_Image_Constructor.lvclass">)
              n393 = call "Read Save Image.lvclass.vi"("error in (no error)"=w944, "Image Constructor in"=w945) -> ("error out"=w947:errorcluster, "Save Image.lvclass"=w946:refnum<class "Save Image.lvclass">)  [unwired: 7 in, 1 out]
              n394 = call "Read Image Information.vi"("error in (no error)"=w947, "Save Image in"=w946) -> ("error out"=w949:errorcluster, "Image Information"=w950:T6)  [unwired: 7 in, 1 out]
              n395 = Unbundle By Name(w950) -> ("Base Name"=w948:string)
            }
            frame "OBSERVATION_TITLE" {
              n396 = Unbundle By Name(w958) -> ("Simulated_Image_Constructor.lvclass"=w953:refnum<class "Simulated_Image_Constructor.lvclass">)
              n397 = call "Read Save Image.lvclass.vi"("error in (no error)"=w952, "Image Constructor in"=w953) -> ("error out"=w955:errorcluster, "Save Image.lvclass"=w954:refnum<class "Save Image.lvclass">)  [unwired: 7 in, 1 out]
              n398 = call "Read Observation Title.vi"("error in (no error)"=w955, "Save Image in"=w954) -> ("error out"=w957:errorcluster, "OBS_TITLE.Value"=w956:string)  [unwired: 7 in, 1 out]
            }
            frame "COMMENT" {
              n399 = Unbundle By Name(w965) -> ("Simulated_Image_Constructor.lvclass"=w960:refnum<class "Simulated_Image_Constructor.lvclass">)
              n400 = call "Read Save Image.lvclass.vi"("error in (no error)"=w959, "Image Constructor in"=w960) -> ("error out"=w962:errorcluster, "Save Image.lvclass"=w961:refnum<class "Save Image.lvclass">)  [unwired: 7 in, 1 out]
              n401 = call "Read Comment.vi"("error in (no error)"=w962, "Save Image in"=w961) -> ("error out"=w964:errorcluster, "COMMENT.Value"=w963:string)  [unwired: 7 in, 1 out]
            }
            frame "TEMPERATURE" {
              n402 = Unbundle By Name(w973) -> ("Simulated_Image_Constructor.lvclass"=w967:refnum<class "Simulated_Image_Constructor.lvclass">)
              n403 = call "Read Simulated_CCD_Camera.lvclass.vi"("error in (no error)"=w966, "Image Constructor in"=w967) -> ("error out"=w969:errorcluster, "Simulated_CCD_Camera.lvclass"=w968:refnum<class "Simulated_CCD_Camera.lvclass">)  [unwired: 7 in, 1 out]
              n404 = call "Read Temperature.vi"("error in (no error)"=w969, "CCDCamera in"=w968) -> ("error out"=w971:errorcluster, "Temperature"=w972:i32)  [unwired: 7 in, 1 out]
              n405 = Number To Decimal String(number=w972) -> (decimal integer string=w970:string)  [unwired: 1 in]
            }
            frame "SHUTTER" {
              n406 = Unbundle By Name(w981) -> ("Simulated_Image_Constructor.lvclass"=w975:refnum<class "Simulated_Image_Constructor.lvclass">)
              n407 = call "Read Simulated_CCD_Camera.lvclass.vi"("error in (no error)"=w974, "Image Constructor in"=w975) -> ("error out"=w977:errorcluster, "Simulated_CCD_Camera.lvclass"=w976:refnum<class "Simulated_CCD_Camera.lvclass">)  [unwired: 7 in, 1 out]
              n408 = call "Read Shutter Mode.vi"("error in (no error)"=w977, "CCDCamera in"=w976) -> ("error out"=w979:errorcluster, "Shutter Mode"=w980:u8)  [unwired: 7 in, 1 out]
              n409 = Number To Decimal String(number=w980) -> (decimal integer string=w978:string)  [unwired: 1 in]
            }
            frame "PREAMP" {
              n410 = Unbundle By Name(w989) -> ("Simulated_Image_Constructor.lvclass"=w983:refnum<class "Simulated_Image_Constructor.lvclass">)
              n411 = call "Read Simulated_CCD_Camera.lvclass.vi"("error in (no error)"=w982, "Image Constructor in"=w983) -> ("error out"=w985:errorcluster, "Simulated_CCD_Camera.lvclass"=w984:refnum<class "Simulated_CCD_Camera.lvclass">)  [unwired: 7 in, 1 out]
              n412 = call "Read Pre-amp gain.vi"("error in (no error)"=w985, "CCDCamera in"=w984) -> ("error out"=w987:errorcluster, "Pre-amp gain"=w988:u8)  [unwired: 7 in, 1 out]
              n413 = Number To Decimal String(number=w988) -> (decimal integer string=w986:string)  [unwired: 1 in]
            }
            frame "KSERLEN" {
              n414 = Unbundle By Name(w997) -> ("Simulated_Image_Constructor.lvclass"=w991:refnum<class "Simulated_Image_Constructor.lvclass">)
              n415 = call "Read Simulated_CCD_Camera.lvclass.vi"("error in (no error)"=w990, "Image Constructor in"=w991) -> ("error out"=w993:errorcluster, "Simulated_CCD_Camera.lvclass"=w992:refnum<class "Simulated_CCD_Camera.lvclass">)  [unwired: 7 in, 1 out]
              n416 = call "Read Kinetic Series Length.vi"("error in (no error)"=w993, "CCDCamera in"=w992) -> ("error out"=w995:errorcluster, "Kinetic Series Length"=w996:u32)  [unwired: 7 in, 1 out]
              n417 = Number To Decimal String(number=w996) -> (decimal integer string=w994:string)  [unwired: 1 in]
            }
            frame "CUBES" {
              n418 = Unbundle By Name(w1001) -> ("Cubes"=w1000:u16)
              n419 = Number To Decimal String(number=w1000) -> (decimal integer string=w998:string)  [unwired: 1 in]
            }
          }
          n420 = Unbundle By Name(w840) -> ("RxTx.lvclass"=w842:refnum<class "RxTx.lvclass">)
          n421 = call "Send TX Message.vi"("error in (no error)"=w839, "element"=w838, "RxTx in"=w842) -> ("error out"=w832:errorcluster, "RxTx out"=w841:refnum<class "RxTx.lvclass">)  [unwired: 7 in]
          n422 = Bundle By Name(cluster=w840, "RxTx.lvclass"=w841) -> (w831:refnum<class "Channel.lvclass">)
          n423 = Unbundle By Name(w831) -> ("State Machine.lvclass"=w833:refnum<class "State Machine.lvclass">)
          n424 = call-dynamic "Write State.vi"("error in (no error)"=w832, "State"="False", "State Machine in"=w833) -> ("error out"=w829:errorcluster, "State Machine out"=w835:refnum<class "State Machine.lvclass">)  [unwired: 7 in]
          n425 = Bundle By Name(cluster=w831, "State Machine.lvclass"=w835) -> (w830:refnum<class "Channel.lvclass">)
        }
        frame "INIT" {
          n426 = Unbundle By Name(w1033) -> ("Simulated_Image_Constructor.lvclass"=w1018:refnum<class "Simulated_Image_Constructor.lvclass">)
          n427 = call "Read Simulated_CCD_Camera.lvclass.vi"("error in (no error)"=w1017, "Image Constructor in"=w1018) -> ("error out"=w1015:errorcluster, "Simulated_CCD_Camera.lvclass"=w1016:refnum<class "Simulated_CCD_Camera.lvclass">, "Image Constructor out"=w1013:refnum<class "Simulated_Image_Constructor.lvclass">)  [unwired: 7 in]
          n428 = call-dynamic "Initialize Camera.vi"("error in (no error)"=w1015, "CCDCamera in"=w1016) -> ("error out"=w1025:errorcluster, "CCDCamera out"=w1026:refnum<class "Simulated_CCD_Camera.lvclass">)  [unwired: 8 in]
          n429 = call "Standard Setup.vi"("error in (no error)"=w1025, "CCDCamera in"=w1026) -> ("error out"=w1020:errorcluster, "CCDCamera out"=w1021:refnum<class "Simulated_CCD_Camera.lvclass">)  [unwired: 8 in]
          n430 = call-dynamic "Set Camera Configuration.vi"("error in (no error)"=w1020, "CCDCamera in"=w1021) -> ("error out"=w1023:errorcluster, "CCDCamera out"=w1024:refnum<class "Simulated_CCD_Camera.lvclass">)  [unwired: 8 in]
          n431 = call-dynamic "Write Tempo de espera.vi"("error in (no error)"=w1023, "Tempo de espera"=u16 30, "CCDCamera in"=w1024) -> ("error out"=w1002:errorcluster, "CCDCamera out"=w1014:refnum<class "Simulated_CCD_Camera.lvclass">)  [unwired: 7 in]
          n432 = call "Write Simulated_CCD_Camera.lvclass.vi"("error in (no error)"=w1002, "Simulated_CCD_Camera.lvclass"=w1014, "Image Constructor in"=w1013) -> ("error out"=w1012:errorcluster, "Image Constructor out"=w1011:refnum<class "Simulated_Image_Constructor.lvclass">)  [unwired: 7 in]
          n433 = call "Read Save Image.lvclass.vi"("error in (no error)"=w1012, "Image Constructor in"=w1011) -> ("error out"=w1005:errorcluster, "Save Image.lvclass"=w1008:refnum<class "Save Image.lvclass">, "Image Constructor out"=w1006:refnum<class "Simulated_Image_Constructor.lvclass">)  [unwired: 7 in]
          n434 = call "Write Image Path.vi"("error in (no error)"=w1005, "Image Path"="../../Today/", "Save Image in"=w1008) -> ("error out"=w1004:errorcluster, "Save Image out"=w1007:refnum<class "Save Image.lvclass">)  [unwired: 7 in]
          n435 = call "Write Save Image.lvclass.vi"("error in (no error)"=w1004, "Save Image.lvclass"=w1007, "Image Constructor in"=w1006) -> ("error out"=w1009:errorcluster, "Image Constructor out"=w1010:refnum<class "Simulated_Image_Constructor.lvclass">)  [unwired: 7 in]
          n436 = Bundle By Name(cluster=w1033, "Cubes"=u16 1 ("#sequences"), "Simulated_Image_Constructor.lvclass"=w1010) -> (w1032:refnum<class "Channel.lvclass">)
          n437 = Unbundle By Name(w1032) -> ("State Machine.lvclass"=w1029:refnum<class "State Machine.lvclass">)
          n438 = call-dynamic "Write State.vi"("error in (no error)"=w1009, "State"="False", "State Machine in"=w1029) -> ("error out"=w1027:errorcluster, "State Machine out"=w1031:refnum<class "State Machine.lvclass">)  [unwired: 7 in]
          n439 = Bundle By Name(cluster=w1032, "State Machine.lvclass"=w1031) -> (w1028:refnum<class "Channel.lvclass">)
        }
      }
    }
    frame Error {
    }
  }
  "error out" <- w3
  "Channel out" <- w1
